vi "Controls.vi"() -> ()   [LabVIEW 2013]
uses:
  openfpgaref.8.6.ctl
  <vilib>/rvi/interface/nirviReadWriteControl/nirviReadWriteControl.xnode
  NiFpgaLv.dll
  <vilib>/Utility/error.llb/Error Cluster From Error Code.vi
  FPGA Bitfiles/UHR-FleezersInst_FPGATarget_UHR-Fleezers_Leonardo042018V4.lvbitx
  <vilib>/rvi/errors/niLvFpgaAdjustHostInterfaceError.vi
  <vilib>/gmath/NI_Gmath.lvlib
  <vilib>/gmath/statdist.llb/Exp Random.vi
  <vilib>/gmath/statdist.llb/Gamma Random.vi
  <vilib>/Platform/TimedLoop/XDataNode/wakeup.ctl
  <vilib>/Platform/TimedLoop/XDataNode/XDNodeRunTimeDep.lvlib
  <vilib>/Platform/TimedLoop/XDataNode/nitl_modes.ctl
  <vilib>/Platform/TimedLoop/XDataNode/timing_clust.ctl
  <vilib>/Platform/TimedLoop/XDataNode/XDataNode.xnode
  <vilib>/Utility/miscctls.llb/LVMinMaxIncTypeDef.ctl
panel:
  out "Current MCL (V)":dbl=5.657514378627918
  out "B factor":dbl=0.9916156324677038
  in  "Setpoint offset\nCorrection values":dbl[](array[numeric])=[0.024496601698410773, 0.024671186719617436, 0.024845771740824106, 0.025020356762030765, 0.02519494178323743, 0.025369526804444095, 0.025544111825650764, 0.025718696846857424, 0.025893281868064093, 0.026067866889270756, 0.026242451910477423, 0.026417036931684082, 0.02659162195289075, 0.026766206974097418, 0.02694079199530408, 0.027115377016510744, 0.027289962037717407, 0.027464547058924076, 0.02763913208013074, 0.027813717101337402, 0.027988302122544065, 0.02816288714375073, 0.028337472164957394, 0.02851205718616406, 0.028686642207370723, 0.028861227228577393, 0.02903581224978405, 0.029210397270990722, 0.029384982292197385, 0.02955956731340405, 0.02973415233461071, 0.029908737355817377, 0.030083322377024047, 0.03025790739823071, 0.030432492419437372, 0.030607077440644035, 0.0307816624618507, 0.030956247483057368, 0.03113083250426403, 0.0313054175254707, 0.03148000254667736, 0.03165458756788402, 0.03182917258909068, 0.03200375761029735, 0.032178342631504014, 0.03235292765271068, 0.03252751267391735, 0.03270209769512401, 0.03287668271633068, 0.033051267737537346, 0.033225852758744005, 0.03340043777995067, 0.03357502280115733, 0.033749607822364, 0.033924192843570664, 0.03409877786477733, 0.034273362885983996, 0.034447947907190656, 0.03462253292839732, 0.03479711794960398, 0.03497170297081065, 0.035146287992017314, 0.03532087301322398, 0.035495458034430646, 0.035670043055637306, 0.03584462807684397, 0.036019213098050645, 0.036193798119257305, 0.03636838314046397, 0.03654296816167063, 0.0367175531828773, 0.03689213820408396, 0.03706672322529063, 0.037241308246497296, 0.037415893267703955, 0.03759047828891062, 0.03776506331011729, 0.03793964833132395, 0.03811423335253061, 0.03828881837373728, 0.038463403394943946, 0.038637988416150605, 0.03881257343735727, 0.03898715845856393, 0.0391617434797706, 0.03933632850097726, 0.03951091352218393, 0.039685498543390596, 0.03986008356459726, 0.04003466858580393, 0.040209253607010595, 0.040383838628217254, 0.04055842364942392, 0.04073300867063058, 0.040907593691837246, 0.04108217871304391, 0.04125676373425058, 0.041431348755457245, 0.0416059337766639, 0.041780518797870564, 0.04195510381907723, 0.042129688840283896, 0.04230427386149057, 0.04247885888269723, 0.042653443903903895, 0.04282802892511056, 0.04300261394631722, 0.04317719896752389, 0.043351783988730554, 0.04352636900993721, 0.04370095403114388, 0.043875539052350546, 0.04405012407355721, 0.04422470909476388, 0.04439929411597054, 0.044573879137177204, 0.04474846415838387, 0.044923049179590537, 0.045097634200797196, 0.04527221922200386, 0.04544680424321053, 0.045621389264417195, 0.04579597428562386, 0.04597055930683052, 0.04614514432803718, 0.046319729349243846, 0.04649431437045051, 0.04666889939165718, 0.046843484412863845, 0.04701806943407051, 0.04719256456184452, 0.04736536676840916, 0.04753446267808822, 0.047696991448649737, 0.04784953848765512, 0.04799284096907562, 0.048127712917801824, 0.048257934523222495, 0.04838705366421733, 0.04851995197559876, 0.04865949840047511, 0.04880178465045004, 0.0489357994772595, 0.04905304538798107, 0.0491519464532862, 0.049234486275402736, 0.04930263064515607, 0.04935733149089569, 0.04939552771001872, 0.04941451823245213, 0.04941830757306315, 0.049410747020732684, 0.049392795273013504, 0.049367258833286985, 0.049339629147657244, 0.049311849604908836, 0.04928407006216041, 0.049256290519411994, 0.04922851097666357, 0.04920073143391515, 0.04917295189116673, 0.04914517234841831, 0.049117392805669895, 0.049089613262921473, 0.04906183372017306, 0.04903405417742463, 0.04900627463467622, 0.0489784950919278, 0.048950715549179374, 0.04892293600643097, 0.04889515646368254, 0.048867376920934125, 0.0488395973781857, 0.04881181783543728, 0.04878403829268886, 0.04875625874994044, 0.048728479207192026, 0.0487006996644436, 0.04867292012169519, 0.04864514057894676, 0.04861736103619835, 0.048589581493449926, 0.048561801950701505, 0.04853402240795309, 0.04850624286520466, 0.04847846332245625, 0.04845068377970783, 0.04842290423695941, 0.048395124694210985, 0.04836734515146257, 0.04833956560871415, 0.04831178606596573, 0.048284006523217314, 0.048256226980468886, 0.04822844743772048, 0.04820066789497206, 0.048172888352223636, 0.048145108809475215, 0.048117329266726794, 0.04808954972397837, 0.04806177018122996, 0.048033990638481544, 0.048006211095733116, 0.0479784315529847, 0.04795065201023628, 0.04792287246748786, 0.04789509292473944, 0.04786731338199102, 0.0478395338392426, 0.04781175429649418, 0.04778397475374576, 0.047756195210997346, 0.047728415668248925, 0.047700636125500503, 0.04767285658275208, 0.04764507704000366, 0.04761729749725524, 0.047589517954506826, 0.047561738411758404, 0.04753395886900998, 0.04750617932626157, 0.04747839978351315, 0.047450620240764727, 0.047422840698016305, 0.047395061155267884, 0.04736728161251948, 0.047339502069771056, 0.047311722527022634, 0.04728394298427421, 0.04725616344152579, 0.04722838389877737, 0.047200604356028956, 0.047172824813280535, 0.047145045270532114, 0.0471172657277837, 0.04708948618503528, 0.04706170664228686, 0.047033927099538436, 0.047006147556790015, 0.0469783680140416, 0.04695058847129318, 0.04692280892854476, 0.046895029385796344, 0.04686724984304792, 0.0468394703002995, 0.04681169075755108, 0.04678391121480266, 0.04675613167205424, 0.046728352129305824, 0.0467005725865574, 0.04667279304380899, 0.04664501350106057, 0.046617233958312146, 0.046589454415563725, 0.046561674872815303, 0.04653389533006689, 0.046506115787318475, 0.046478336244570054, 0.04645055670182163, 0.04642277715907321, 0.04639499761632479, 0.04636721807357637, 0.046339438530827955, 0.04631165898807953, 0.04628387944533112, 0.0462560999025827, 0.04622832035983428, 0.046200540817085856, 0.046172761274337434, 0.04614498173158901, 0.04611720218884059, 0.04608942264609218, 0.046061643103343757, 0.04603386356059534, 0.04600608401784692, 0.0459783044750985, 0.04595052493235008, 0.04592274538960166, 0.045894965846853236, 0.045867186304104815, 0.0458394067613564, 0.045811627218607986, 0.045783847675859565, 0.045756068133111144, 0.04572828859036272, 0.0457005090476143, 0.04567272950486588, 0.04564494996211747, 0.04561717041936905, 0.04558939087662063, 0.04556161133387221, 0.04553383179112379, 0.04550605224837537, 0.045478272705626946, 0.045450493162878525, 0.04542271362013011, 0.045394934077381696, 0.045367154534633275, 0.045339374991884854, 0.04531159544913643, 0.04528381590638801, 0.04525603636363959, 0.04522825682089117, 0.045200477278142755, 0.045172697735394333, 0.04514491819264592, 0.0451171386498975, 0.04508935910714908, 0.045061579564400656, 0.045033800021652234, 0.04500602047890381, 0.04497824093615539, 0.044950461393406985, 0.04492268185065856, 0.04489490230791014, 0.04486712276516172, 0.0448393432224133, 0.04481156367966488, 0.044783784136916464, 0.04475600459416805, 0.04472822505141963, 0.04470044550867121, 0.044672665965922786, 0.044644886423174365, 0.044617106880425944, 0.04458932733767752, 0.04456154779492911, 0.044533768252180694, 0.04450598870943227, 0.04447820916668385, 0.04445042962393543, 0.04442265008118701, 0.04439487053843859, 0.04436709099569017, 0.04433931145294175, 0.04431153191019333, 0.04428375236744492, 0.044255972824696496, 0.044228193281948075, 0.044200413739199654, 0.04417263419645123, 0.04414485465370281, 0.0441170751109544, 0.04408929556820598, 0.04406151602545756, 0.04403373648270914, 0.04400595693996072, 0.0439781773972123, 0.043950397854463884, 0.04392261831171546, 0.04389483876896704, 0.04386705922621863, 0.043839279683470206, 0.043811500140721785, 0.04378372059797336, 0.04375594105522494, 0.04372816151247652, 0.04370038196972811, 0.04367260242697968, 0.043644822884231264, 0.04361704334148285, 0.04358926379873443, 0.04356148425598601, 0.043533704713237587, 0.043505925170489165, 0.04347814562774075, 0.04345036608499233, 0.043422586542243916, 0.043394806999495494, 0.04336702745674707, 0.04333924791399865, 0.04331146837125023, 0.043283688828501816, 0.0432559092857534, 0.04322812974300498, 0.04320035020025656, 0.04317257065750814, 0.04314479111475972, 0.043117011572011296, 0.04308923202926288, 0.04306145248651446, 0.04303367294376604, 0.043005893401017625, 0.0429781138582692, 0.04295033431552078, 0.04292255477277236, 0.04289477523002394, 0.04286699568727552, 0.0428392161445271, 0.042811436601778684, 0.04278365705903027, 0.04275587751628185, 0.04272809797353343, 0.042700318430785006, 0.042672538888036585, 0.042644759345288163, 0.04261697980253975, 0.04258920025979133, 0.04256142071704291, 0.04253364117429449, 0.04250586163154607, 0.04247808208879765, 0.04245030254604923, 0.04242252300330081, 0.042394743460552387, 0.04236696391780398, 0.04233918437505556, 0.04231140483230714, 0.042283625289558716, 0.042255845746810294, 0.04222806620406188, 0.04220028666131346, 0.04217250711856504, 0.042144727575816616, 0.0421169480330682, 0.04208916849031978, 0.04206138894757136, 0.04203360940482294, 0.04200582986207452, 0.0419780503193261, 0.041950270776577675, 0.04192249123382926, 0.041894711691080846, 0.041866932148332425, 0.041839152605584004, 0.04181137306283558, 0.04178359352008716, 0.04175581397733874, 0.04172803443459032, 0.0417002548918419, 0.04167247534909349, 0.04164469580634507, 0.04161691626359665, 0.04158913672084823, 0.041561357178099806, 0.0415335776353514, 0.04150579809260298, 0.041478018549854556, 0.041450239007106135, 0.041422459464357714, 0.04139467992160929, 0.04136690037886087, 0.04133912083611246, 0.04131134129336403, 0.04128356175061562, 0.04125578220786719, 0.04122800266511878, 0.04120022312237036, 0.04117244357962194, 0.041144664036873516, 0.041116884494125094, 0.04108910495137668, 0.04106132540862826, 0.04103354586587984, 0.041005766323131417, 0.040977986780383, 0.04095020723763458, 0.04092242769488616, 0.04089464815213774, 0.04086686860938932, 0.0408390890666409, 0.04081130952389249, 0.04078352998114407, 0.040755750438395646, 0.040727970895647225, 0.040700191352898804, 0.04067241181015039, 0.040644632267401976, 0.04061685272465355, 0.04058907318190513, 0.04056129363915671, 0.04053351409640829, 0.04050573455365987, 0.04047795501091145, 0.040450175468163034, 0.04042239592541461, 0.0403946163826662, 0.04036683683991778, 0.04033905729716935, 0.040311277754420935, 0.040283498211672514, 0.0402557186689241, 0.04022793912617567, 0.04020015958342725, 0.040172380040678836, 0.04014460049793042, 0.040116820955182, 0.04008904141243358, 0.04006126186968516, 0.04003348232693674, 0.04000570278418832, 0.03997792324143991, 0.03995014369869149, 0.039922364155943066, 0.039894584613194645, 0.03986680507044622, 0.0398390255276978, 0.03981124598494939, 0.03978346644220096, 0.039755686899452546]
  in  "Negate offset difference":bool
  in  "Target Force (pN)":dbl=10.5
  out "Trap X (AI1)":T1={"Trap 1"=0.030792236328125, "Trap 2"=-0.011322021484375}
  out "Trap X AI1 (DMA)":T2={"Set 1"=0.030731201171875, "Set 2"=-0.0113525390625}
  in  "Pump 1 contents":string="Top: DNA beads" caption="contents"
  in  "All Pump Parameters":T3={"Pump 1"={"Diameter (mm)"=4.61, "Units"=4.0, "Volume"=100.0, "Rate"=50.0}, "Pump 2"={"Diameter (mm)"=4.61, "Units"=3.0, "Volume"=0.0, "Rate"=0.0}, "Pump 3"={"Diameter (mm)"=4.61, "Units"=4.0, "Volume"=100.0, "Rate"=250.0}}
  in  "Pump write delay (ms)":dbl=300.0
  in  "Save scans":bool=TRUE
  out "MCL Scanning":bool
  in  "T1 alpha_x (nm/V)":dbl=701.8425766517444 step=10.0 format="%#_3g"
  in  "T2 alpha_x (nm/V)":dbl=806.869454518421 step=10.0 format="%#_3g"
  in  "T1 kappa_x (pN/nm)":dbl=0.1608167093260824 min=0.0 step=0.001 format="%#_2g"
  in  "T2 kappa_x (pN/nm)":dbl=0.13871102209446912 min=0.0 step=0.001 format="%#_2g"
  in  "T1 offset_x (mV)":dbl=44.132512662199076 format="%#_2g"
  in  "T2 offset_x (mV)":dbl=-16.403354316809207 format="%#_2g"
  in  "Freq switch delay":u16=9
  in  "Swap F1 and F2":bool
  in  "Amp switch delay":u16=4
  in  "Phase offset method":u8=3
  in  "Phase increment trap 1":fxp<+/-,64,32>
  in  "Phase increment trap 2":fxp<+/-,64,32>
  in  "RF phase reset before cycles":bool
  out "Initial delta (MHz)":dbl=20.0
  in  "AOM X Cal (nm/MHz)":dbl=174.0
  in  "Invert APD Gate":bool caption="Invert Gate"
  in  "APD Gate ON Count":u32=150 caption="Gate ON Count"
  in  "APD Gate OFF Count":u32=450 caption="Gate OFF Count"
  in  "APD Gate":enum32{"ON", "OFF", "Interlace"}(radio)=enum."Interlace"
  in  "APD Integration Time (s)":dbl=0.01 caption="Integration Time (s)"
  in  "APD 1 AO Mult.":i16=1 min=1
  in  "APD 2 AO Mult.":i16=1 min=1
  in  "Phase Adj. (APD Acq)":i16=20
  in  "Phase Adj. (APD 2 Gate)":i16=20
  in  "Phase Adj. (APD 1 Gate)":i16=20
  in  "Green FB Gains":T4={"proportional gain (Kc)"=10, "integral gain (Kc*Ts/Ti)"=5, "derivative gain (Kc*Td/Ts)"=0}
  in  "Current When FB OFF (%)":dbl=10.0 min=0.0 max=100.0 step=1.0
  in  "Green int current ON count adj":u32=150
  in  "Green FB Setpoint (mV)":dbl=100.0
  in  "PID gains":T4={"proportional gain (Kc)"=0, "integral gain (Kc*Ts/Ti)"=5, "derivative gain (Kc*Td/Ts)"=0}
  in  "DIO count 1 (ticks)":u32=200
  in  "DIO count 2 (ticks)":u32=200
  in  "DIO count 3 (ticks)":u32=200
  in  "BD 1 Amplitude 1 (%)":dbl=40.0 min=0.0 max=75.0 step=1.0
  in  "BD 1 Amplitude 2 (%)":dbl=42.0 min=0.0 max=75.0 step=1.0
  in  "BD 1 Amplitude 3 (%)":dbl min=0.0 max=75.0 step=1.0
  in  "BD 2 Amplitude 1 (%)":dbl min=0.0 max=75.0 step=1.0
  in  "BD 2 Amplitude 2 (%)":dbl min=0.0 max=75.0 step=1.0
  in  "BD 2 Amplitude 3 (%)":dbl min=0.0 max=75.0 step=1.0
  out "X RF Amplitude Limits (%)":T5={"Minimum"=0.0, "Maximum"=75.0, "Increment"=1.0}
  out "Y RF Amplitude Limits (%)":T5={"Minimum"=0.0, "Maximum"=75.0, "Increment"=1.0}
  out "Feedback overload":bool
  out "APD 1 Rate (Hz)":dbl format="%#_3p"
  out "AI labels":string[](array[string])=["T1 Y", "T1 X", "T1 Sum", "T2 Y", "T2 X", "T2 Sum", "T1 FB X", "T2 FB Sum", "T2 FB X", "T2 FB Sum", "PSD Y", "PSD X", "PSD Sum"]
  out "Bead Mean (nm)":dbl=13.506045465071283 caption="Mean (nm)" format="%0.2f"
  in  "AI Count (ticks)":u32=200
  in  "N sets to save":u32=200 caption="N Sets"
  out "APD Int. Count":u32=400000 format="%.0p"
  in  "Scale intensities":bool
  in  "Scale factor":dbl=0.25
  in  "MCL Tracking":bool
  out "Zero MCL x position":dbl=5.6547922360429315
  out "Zero T1 position":dbl=70.0
  in  "Read setpoint correction\nfile":bool
  in  "Setpoint correction\noffset file":path
  in  "Raster target force (pN)":dbl=10.0
  in  "Trap Pos FB Int Count":u16=100
  in  "Trap Pos. FB Out Scale 2^n":u8=23 caption="Action Scale"
  in  "Set SP to Reading":bool
  in  "Set SP Using...":bool
  in  "Simulate stepping":bool
  in  "Step size (nm)":dbl min=0.0
  in  "Backtrack probability":dbl min=0.0 max=1.0
  in  "Mean dwell time (s)":dbl=0.001 min=0.001
  in  "Distribution":enum16{"uniform", "Exponential", "Gamma2"}(ring)
  out "Step taken":dbl
  in  "Number of steps":i32
  out "Step duration":dbl
  in  "Trap Pos FB SP":fxp<+/-,16,1>=0.231353759765625 caption="Setpoint"
  in  "Trap Pos. FB Range":T6={"output high"=0.999969482421875, "output low"=-1.0}
  in  "Trap Pos. FB Gains":T7={"proportional gain (Kc)"=20.0, "integral gain (Kc*Ts/Ti)"=3.0, "derivative gain (Kc*Td/Ts)"=0.0} {"proportional gain (Kc)" format="%.11g"; "integral gain (Kc*Ts/Ti)" format="%.11g"; "derivative gain (Kc*Td/Ts)" format="%.11g"}
  in  "Trap Pos. FB Mult Factor":i64=8388608
  in  "Trap Pos. FB Offset Factor":i64
  in  "Trap Pos FB Negate Action":bool=TRUE
  in  "Trap Pos FB Monitor\nT1 or T2":bool
  in  "Trap Pos. AI1 X Pre-scale":u16
  in  "Diff. FB.":bool=TRUE
  in  "Negate Diff?":bool
  in  "Trap Pos. FB ON":bool
  in  "Reset Trap Pos. FB":bool
  out "Pump 1 cont disp":string="Right: DNA beads "
  out "Pump 3 cont disp":string="Left: ADig beads"
  in  "Flip Green Filter":bool
  in  "Shunt:":bool
  in  "Inject Bottom":bool
  in  "Flush Center Ch Volume (uL)":dbl=15.0
  in  "Flush Center Ch Rate (ul/m)":dbl=100.0
  in  "Total Volume\nFlushed (uL)":dbl
  in  "Inject Valve B":bool caption="Inject Pump 2\n(Flush Center)"
  in  "Ch 3 Inject Volume (uL)":dbl=100.0
  in  "Ch 3 Inject Rate (ul/h)":dbl=250.0
  in  "Pump 3 contents":string="Bottom: ADig beads" caption="contents"
  in  "Chemyx Syringe Pump Serial Port":refnum<visa-resource-name>="ASRL3::INSTR"
  in  "Main:":bool caption="Inject Pump 3"
  in  "Ch 2 Inject Volume (uL)":dbl=100.0
  in  "Ch 1 Inject Rate (ul/h)":dbl=50.0
  in  "Pump pause delay (ms)":u32
  in  "Inject Top:":bool caption="Inject Pump 1"
  in  "Index":dbl=43.0 caption="Save File Index" min=1.0 step=1.0
  out "Save file name":path=path "I:/Data/160525/160525_043.dat"
  out "Save index":dbl=43.0
  in  "Continuous AOD Scanning":bool caption="Continuous Scanning"
  in  "Abort AOD Scan":bool caption="Abort Scan"
  in  "Phase adjust (MCL)":i16 caption="Phase adjust"
  in  "- phase (MCL)":bool
  in  "+ phase (MCL)":bool
  in  "Update Count (MCL)":u32=600
  in  "Abort MCL Scan":bool
  out "Read cal error":errorcluster
  in  "Read Cal":bool
  out "Offset file step size":dbl=0.1
  in  "Offset Values":T8={"Trap 1X offset"=array[500 elements], "Trap 2X offset"=array[500 elements]}
  in  "Auto read offset\ncorrection":bool=TRUE
  out "Data points/scan (f+b)":dbl=240.0 caption="points/scan (f+b)"
  out "Data points/scans (MCL)":dbl=4800.0 caption="Data points/scans"
  in  "Number of scans (MCL)":u64=1 caption="Scans"
  out "Cycles/step (MCL)":u64=2000 caption="Cycles/step" format="%.0p"
  out "N sets should be saved (MCL)":dbl=160.0 caption="N sets should be saved"
  out "Time/f+b scan (s) (MCL)":dbl=2.4 caption="Time/scan (s)"
  out "Desired Scan Incr (V)":dbl=0.14102564102564102
  out "Actual Incr. int (MCL)":i16=462 caption="Incr. int"
  out "Desired incr (int)":dbl=462.098717948718
  in  "N APD Samp/step":dbl=3.0
  in  "Scan Range (V)\n(of steps)":dbl=3.5
  in  "2D or 1D Scan":bool=TRUE
  in  "Fast Scan Dir":bool=TRUE
  in  "Continuous MCL Scanning":bool caption="Cont. Scanning"
  out "Total Time (s) 2":dbl=48.0
  out "Scan steps (AOD)":u64=2000
  out "Data points/scan (f/b)":dbl=2664000.0
  out "Data points/scans":dbl=2664000.0
  in  "Number of F/B Scans (AOD)":u16=1 min=1
  out "Cycles/step (AOD)":u64=666 format="%.3p"
  out "N sets should be saved":dbl=133.2
  out "Time/Scan (s) (AOD)":dbl=19.98 format="%#_2p"
  out "Scan Increment (MHz)":dbl=-0.0050025012506253125
  out "Incr. int (AOD)":i64=-5670036101
  out "Scan Range (MHz)":dbl=-10.0
  out "Final freq. (MHz)":dbl=60.0
  in  "Scan BD":bool=TRUE
  out "Initial freq. (MHz)":dbl=70.0
  out "Final delta (MHz)":dbl=30.0
  out "Final sep (nm)":dbl=1590.0
  out "Initial sep (nm)":dbl=360.0
  in  "Step Size (nm)":dbl=1.0
  in  "Scan Range (nm)":dbl=1683.3000000000002
  in  "Trap 2 Bead Size (nm)":dbl=2100.0
  in  "Trap 1 Bead Size (nm)":dbl=2100.0
  in  "Scan Speed (nm/s)":dbl=100.0
  out "Time to Finish All (min)":dbl=0.666 format="%#_2p"
  in  "GI Frequency, ON count":u32=150 min=1 step=1
  in  "Green FB Count":u32=600
  in  "GI Frequency, OFF count":u32=450 min=1 step=1
  out "APD Acq Rate (Hz)":dbl=100.0 caption="Rate (Hz)"
  in  "+ phase (Green FB)":bool
  in  "- phase (Green FB)":bool
  in  "Phase adj. (Green FB)":i16=10
  in  "Phase adj. (GI) 2":i16=20
  in  "+ phase (GI) 2":bool
  in  "- phase (GI) 2":bool
  in  "+ phase (GI)":bool
  in  "- phase (GI)":bool
  in  "Phase adj. (GI)":i16=5
  in  "+ phase (APD Acq)":bool
  in  "- phase (APD Acq)":bool
  in  "- phase (APD 2 Gate)":bool
  in  "+ phase (APD 2 Gate)":bool
  in  "- phase (APD 1 Gate)":bool
  in  "+ phase (APD 1 Gate)":bool
  in  "Invert GI":bool
  in  "AI2 to Setpoint":cluster{"Set 1":bool, "Set 2":bool}
  in  "Trap Intensity\nSetpoints (V)":cluster{"Set 1":dbl, "Set 2":dbl}={"Set 1"=5.0, "Set 2"=5.0}
  out "AI2 (V)":cluster{"Set 1":dbl, "Set 2":dbl}={"Set 1"=3.087557603686636, "Set 2"=2.914212469862972}
  in  "Reset Feedback":cluster{"Set 1":bool, "Set 2":bool}
  in  "Interlace":bool=TRUE
  in  "Number Interlace Sets":u8=3 min=1 max=3
  in  "Not-Interlacing Set":enum32{"Set 1", "Set 2", "Set 3"}(radio)
  out "Total Counts (ticks)":u32=600
  in  "Trap 1 (ON/OFF)":bool=TRUE
  in  "Trap 2 (ON/OFF)":bool=TRUE
  in  "Saved AOD Raster Scan Parameter Sets":T9(array[cluster])=[{"Scan Range AOD (nm) 2"=500.0, "Step Size AOD (nm) 2"=1.0, "Scan Speed AOD (nm/s) 2"=100.0, "Number of scans (AOD) 2"=1, "Label"="offset curve"}, {"Scan Range AOD (nm) 2"=1000.0, "Step Size AOD (nm) 2"=1.0, "Scan Speed AOD (nm/s) 2"=100.0, "Number of scans (AOD) 2"=1, "Label"="hp raster check"}, {"Scan Range AOD (nm) 2"=6.8, "Step Size AOD (nm) 2"=0.34, "Scan Speed AOD (nm/s) 2"=0.34, "Number of scans (AOD) 2"=1, "Label"="3.4 kbp - 1 bp steps"}]
  in  "Load parameters":bool
  in  "Trap 1 ON":bool=TRUE
  in  "Trap 2 ON":bool=TRUE
  in  "Trap 3 ON":bool
  in  "Trap ON/OFF X or Y Amp?":bool=TRUE
  in  "Feedback On/Off":cluster{"Set 1":bool, "Set 2":bool}={"Set 1"=TRUE, "Set 2"=TRUE}
  in  "All FB On/Off":bool
  in  "Delayed Interlace Start":bool
  in  "Delay to Interlace (s)":dbl
  in  "Round T2 X":bool caption="Round"
  in  "Round T1 X":bool caption="Round"
  in  "Oscillate Set 2":bool
  in  "Middle freq for \nsymmetric (MHz)":dbl=78.0
  in  "T2 for asymmetric\n(MHz)":dbl=85.0
  in  "Symmetric manual \ntrap motion":bool
  in  "Dynamic Force FB":bool=TRUE
  in  "Phase adj. (AI1)":i16
  in  "- phase (AI1)":bool
  in  "+ phase (AI1)":bool
  in  "Adjust Scale\nto Mean":bool
  in  "Above (kHz)":dbl=2.0
  in  "Below (kHz)":dbl=0.5
  in  "Rescale on Mean":bool
  in  "Amplitude (nm)":dbl=1.0
  out "AI rate (Hz)":dbl=200000.0 format="%#_6p"
  out "Ave. Rate (Hz)":dbl=200000.0 format="%#_6p"
  out "Ave. Period (s)":dbl=5e-06 format="%#_6p"
  out "Data Rate (Hz)":dbl=66666.66666666667 caption="Trap Data Rate (Hz)" format="%#_3p"
  out "Data Period (s)":dbl=1.4999999999999999e-05 caption="Trap Data Period (s)" format="%#_6p"
  in  "Sets to FIFO (Traps)":T10={"Set 1"=TRUE, "Set 2"=TRUE, "Set 3"=FALSE}
  out "Save Data Rate (Hz)":dbl=133.33333333333334 caption="Rate (Hz)" format="%#_6p"
  out "Save Data Period (s)":dbl=0.0075 caption="Period (s)" format="%#_6p"
  in  "N Acq Sets (Traps + Fl.)":i16=3
  out "# Samples/channel":u32=40000 format="%.0p"
  out "Trap AI Elements/DMA read":u32=320000 format="%.0p"
  out "DMA Update Period (s)":dbl=0.3
  out "APD Samples/FIFO Acq.":dbl=30.0
  out "Total Time (s)":dbl=60.0
  in  "# Samples/trap":u32=20000 format="%.0p"
  out "APD Elements/DMA read":u32=60
  out "Trap Sets":u32=2
  out "FPGA Averaging":bool
  out "Counts/DMA":dbl=12000000.0 format="%#_6p"
  out "Trap Pos Elements/DMA read":u32=120000 format="%.0p"
  out "error out 2":errorcluster
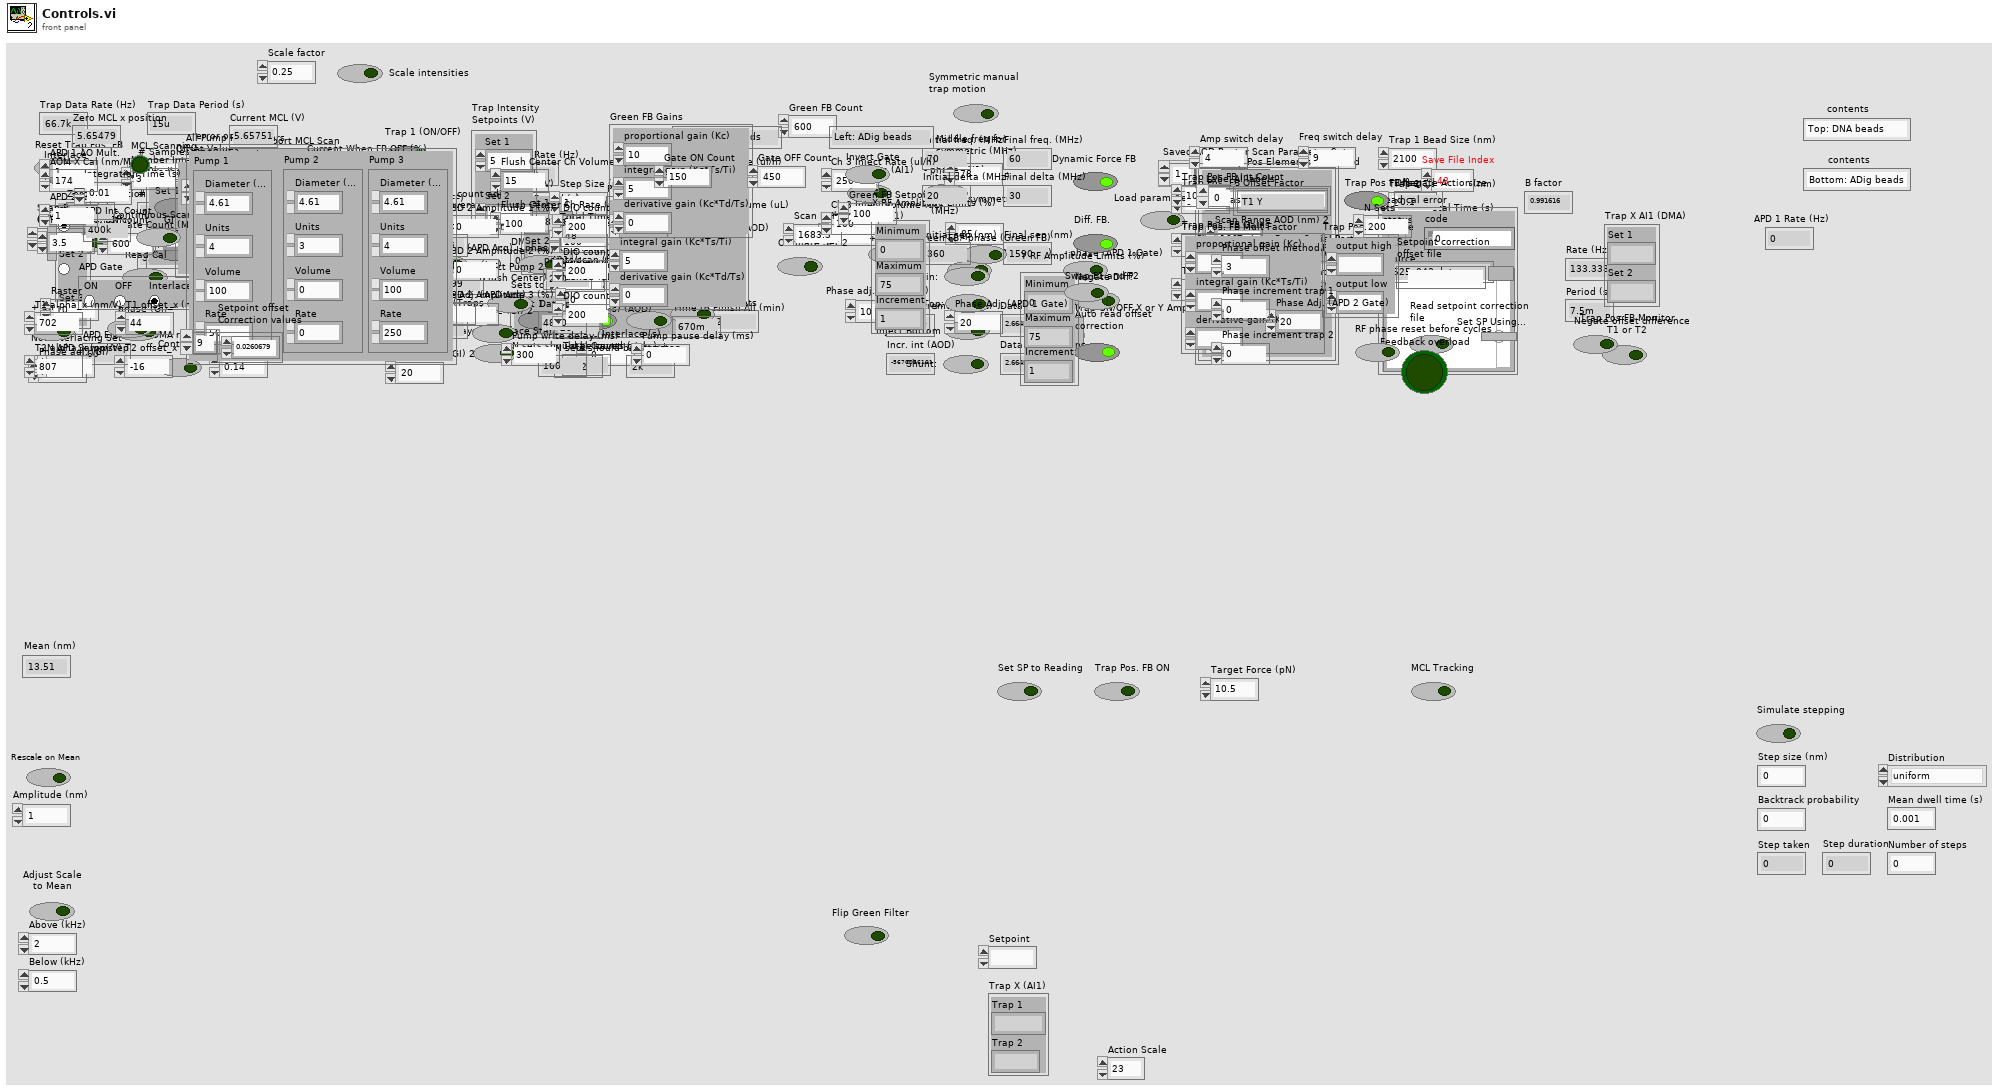
[diagram p1: front panel]
types:
  T1 = cluster{"Trap 1":fxp<+/-,16,1>, "Trap 2":fxp<+/-,16,1>}
  T2 = cluster{"Set 1":fxp<+/-,16,1>, "Set 2":fxp<+/-,16,1>}
  T3 = cluster{"Pump 1":cluster{"Diameter (mm)":dbl, "Units":dbl, "Volume":dbl, "Rate":dbl}, "Pump 2":cluster{"Diameter (mm)":dbl, "Units":dbl, "Volume":dbl, "Rate":dbl}, "Pump 3":cluster{"Diameter (mm)":dbl, "Units":dbl, "Volume":dbl, "Rate":dbl}}
  T4 = cluster{"proportional gain (Kc)":i16, "integral gain (Kc*Ts/Ti)":i16, "derivative gain (Kc*Td/Ts)":i16}
  T5 = typedef "LVMinMaxIncTypeDef.ctl" = cluster{"Minimum":dbl, "Maximum":dbl, "Increment":dbl}
  T6 = cluster{"output high":fxp<+/-,16,1>, "output low":fxp<+/-,16,1>}
  T7 = cluster{"proportional gain (Kc)":fxp<+/-,16,8>, "integral gain (Kc*Ts/Ti)":fxp<+/-,16,8>, "derivative gain (Kc*Td/Ts)":fxp<+/-,16,8>}
  T8 = cluster{"Trap 1X offset":dbl[], "Trap 2X offset":dbl[]}
  T9 = cluster{"Scan Range AOD (nm) 2":dbl, "Step Size AOD (nm) 2":dbl, "Scan Speed AOD (nm/s) 2":dbl, "Number of scans (AOD) 2":u16, "Label":string}[]
  T10 = cluster{"Set 1":bool, "Set 2":bool, "Set 3":bool}
  T11 = typedef "XDNodeRunTimeDep.lvlib/timing_clust.ctl" = cluster{"Expected End [f-1]":u64, "Actual End [f-1]":u64, "Finished Late? [f-1]":bool, "Expected End [i-1]":u64, "Actual End [i-1]":u64, "Finished Late? [i-1]":bool, "Expected Start [i]":u64, "Actual Start [i]":u64, "Expected Start [f]":u64, "Actual Start [f]":u64, "Source Name":string, "Structure Name":string, "Period":i64, "Deadline":i64, "Offset":i64, "Start":i64, "Priority":i32, "Timeout":i32, "Mode":T12, "Wakeup Reason":T13, "Error":errorcluster, "Source Type":string, "Secondary Source Type":string, "Global End Time":u64, "Global Start Time":u64, "Frame Duration":u64, "Iteration Duration":u64, "Assigned CPU":i32, "I/O Scan Engine Mode":u32}
  T12 = typedef "XDNodeRunTimeDep.lvlib/nitl_modes.ctl" = enum32{"No Change", "Process missed periods, maintain original phase", "Discard missed periods, maintain original phase", "Process missed periods, ignore original phase", "Discard missed periods, ignore original phase"}
  T13 = typedef "XDNodeRunTimeDep.lvlib/wakeup.ctl" = enum32{"Normal", "Aborted", "Asynchronous wakeup", "Timing source error", "Timed loop error", "Timeout"}
  T14 = enum16{"CONNECT", "INITIALIZE VALVES", "DISCONNECT", "MOVE VALVE"}
  T15 = enum16{"open", "replace", "create", "open or create", "replace or create", "replace or create with confirmation"}
  T16 = enum16{"big-endian, network order", "native, host order", "little-endian"}
  T17 = typedef "openfpgaref.8.6.ctl" = refnum<k20>
  T18 = cluster{"Scan Range AOD (nm) 2":dbl, "Step Size AOD (nm) 2":dbl, "Scan Speed AOD (nm/s) 2":dbl, "Number of scans (AOD) 2":u16, "Label":string}
  T19 = cluster{"[0]":dbl, "[1]":dbl, "[2]":dbl, "[3]":dbl, "[4]":dbl, "[5]":dbl}
  T20 = cluster{"Diameter (mm)":dbl, "Units":dbl, "Volume":dbl, "Rate":dbl}
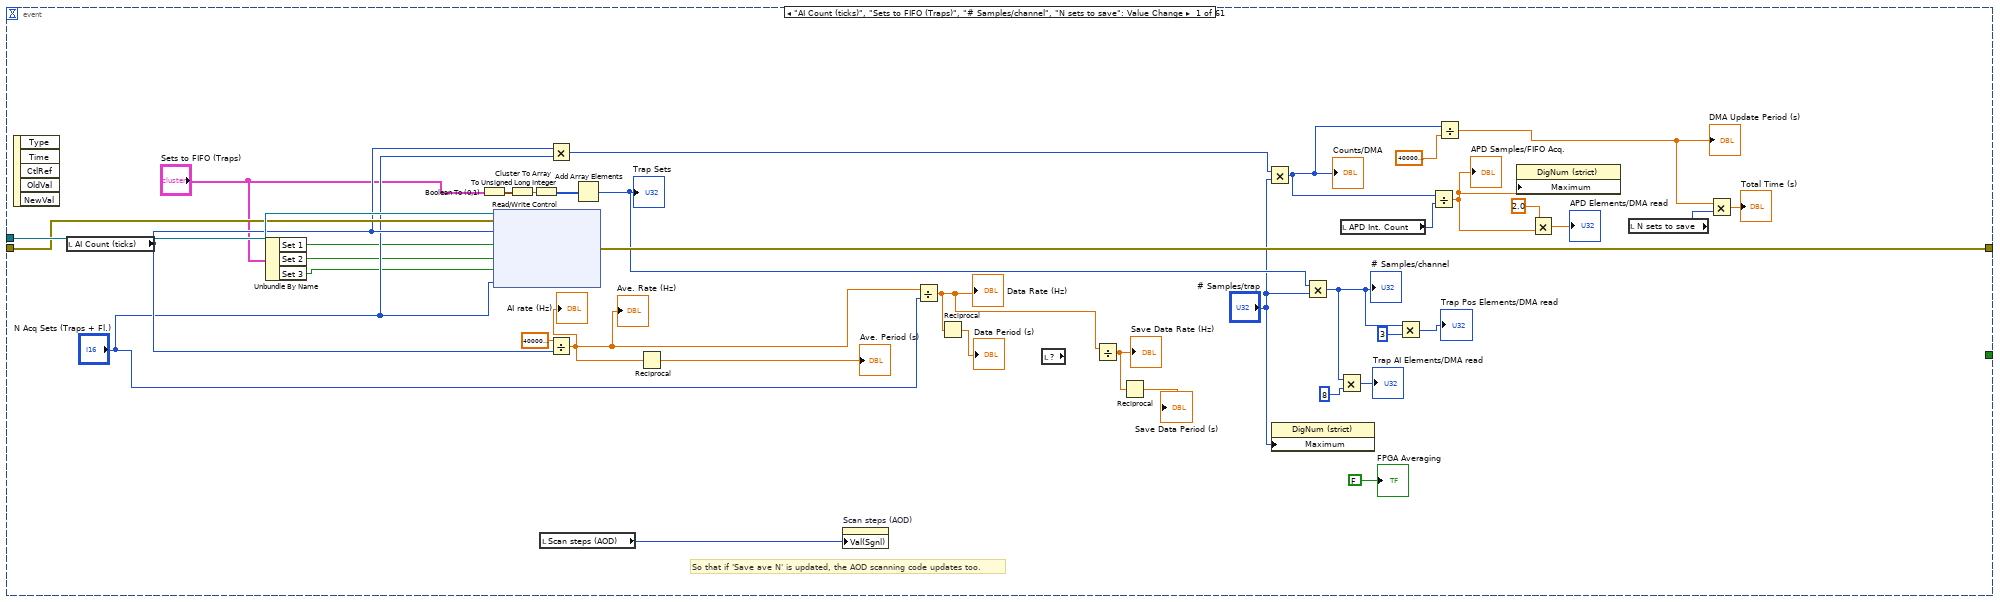
[diagram p2: hidden frame]
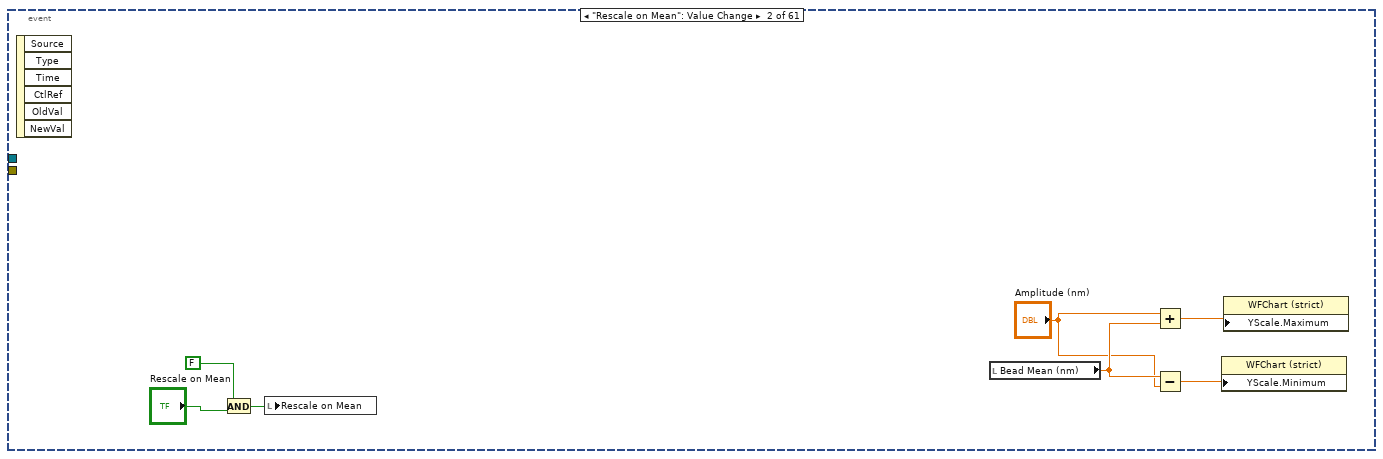
[diagram p3: hidden frame]
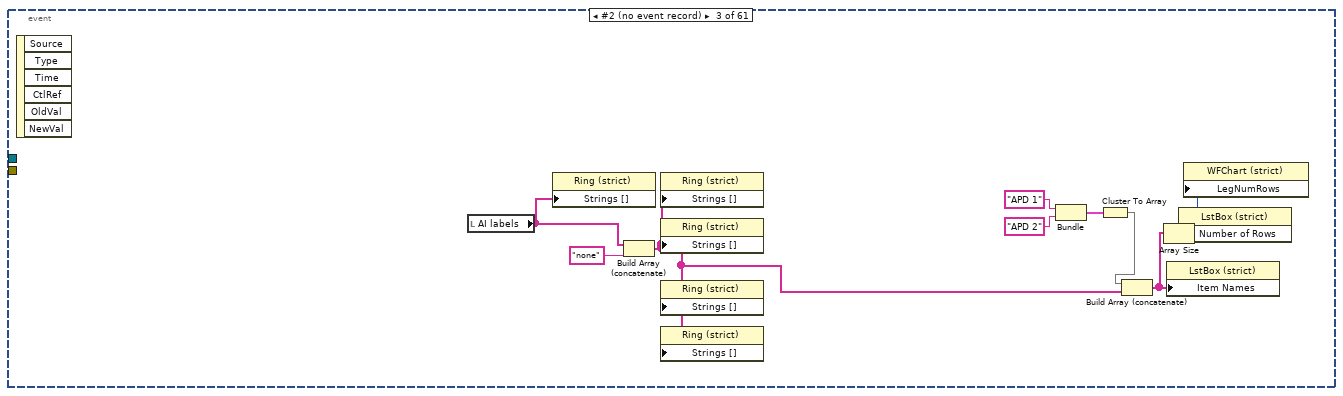
[diagram p4: hidden frame]
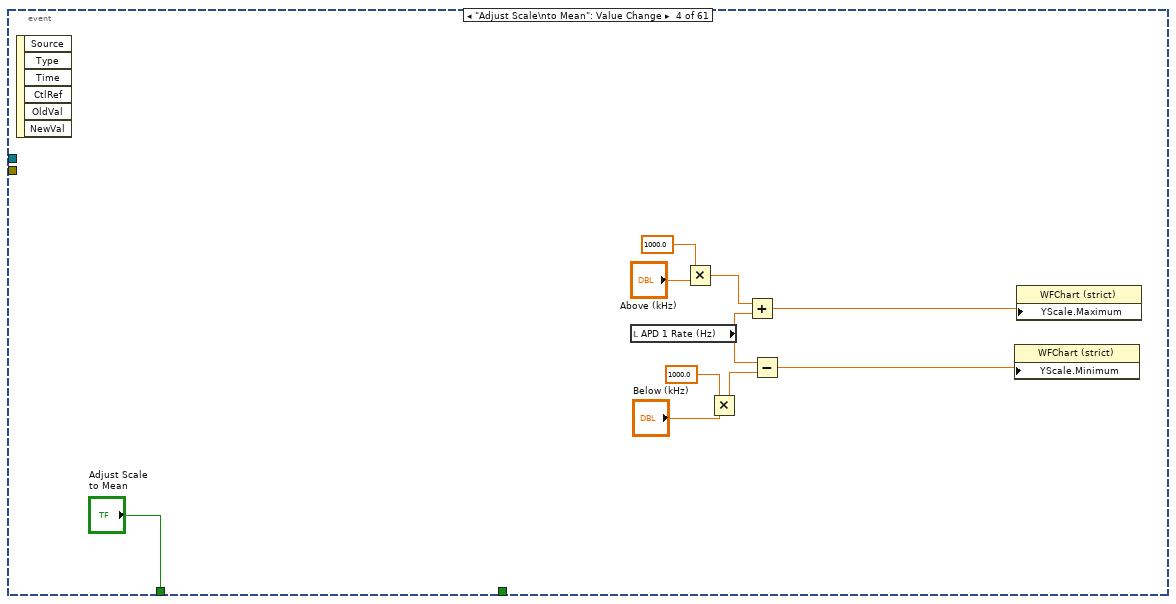
[diagram p5: hidden frame]
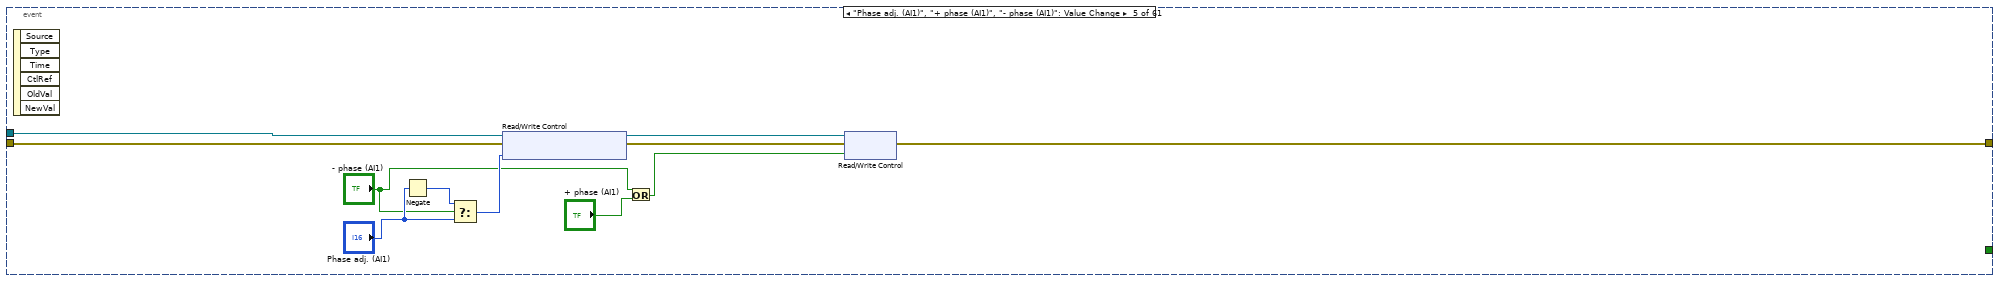
[diagram p6: hidden frame]
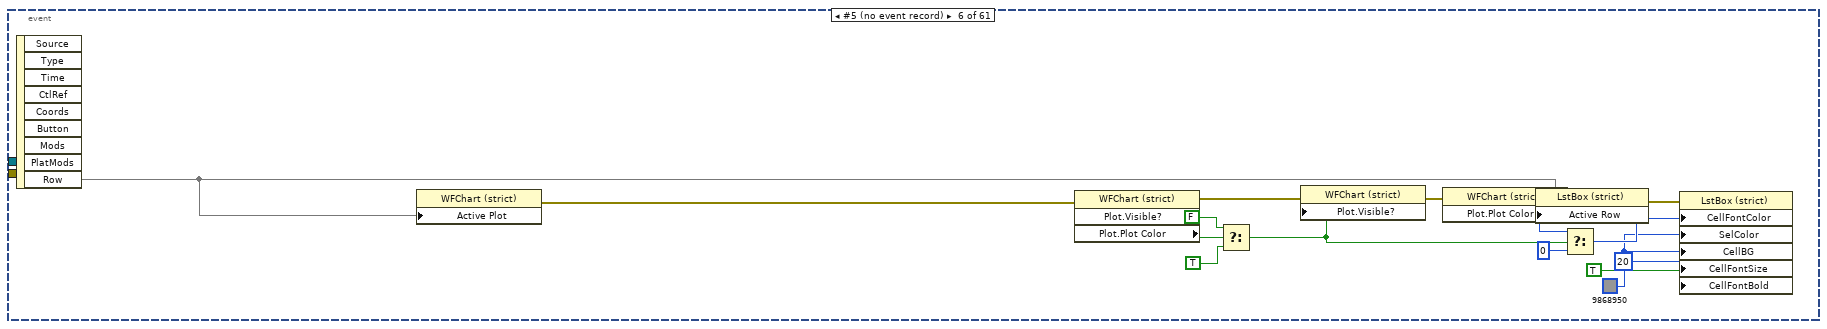
[diagram p7: hidden frame]
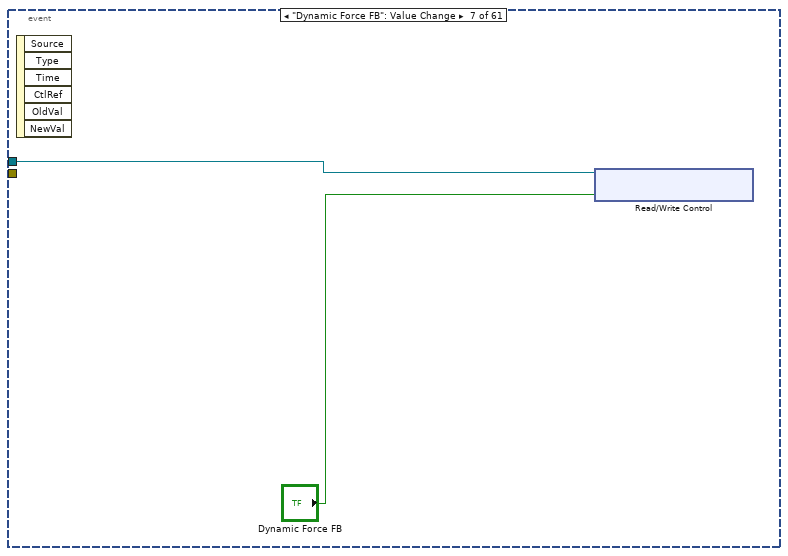
[diagram p8: hidden frame]
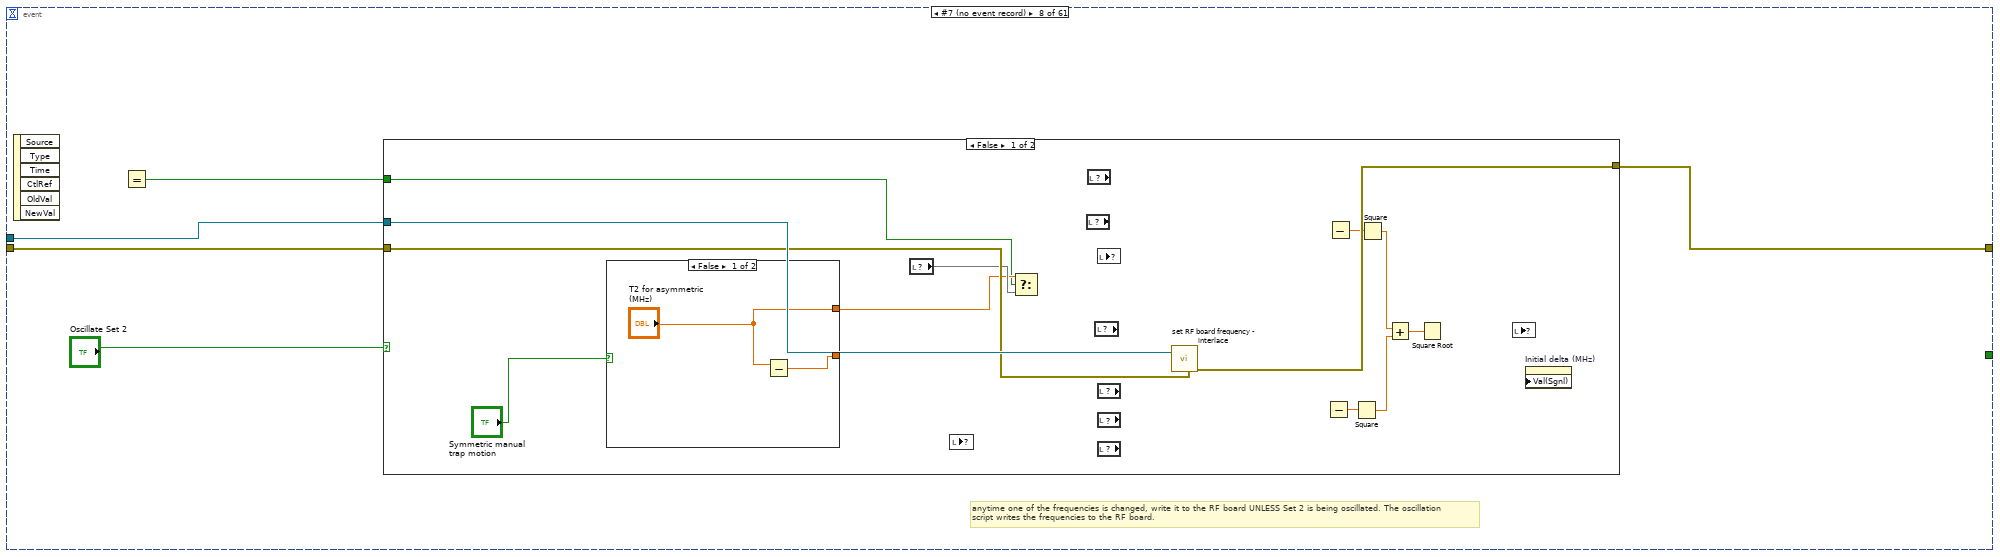
[diagram p9: hidden frame]
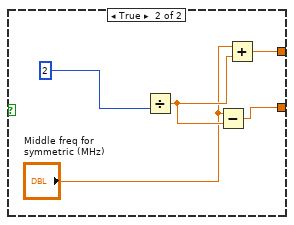
[diagram p10: hidden frame]
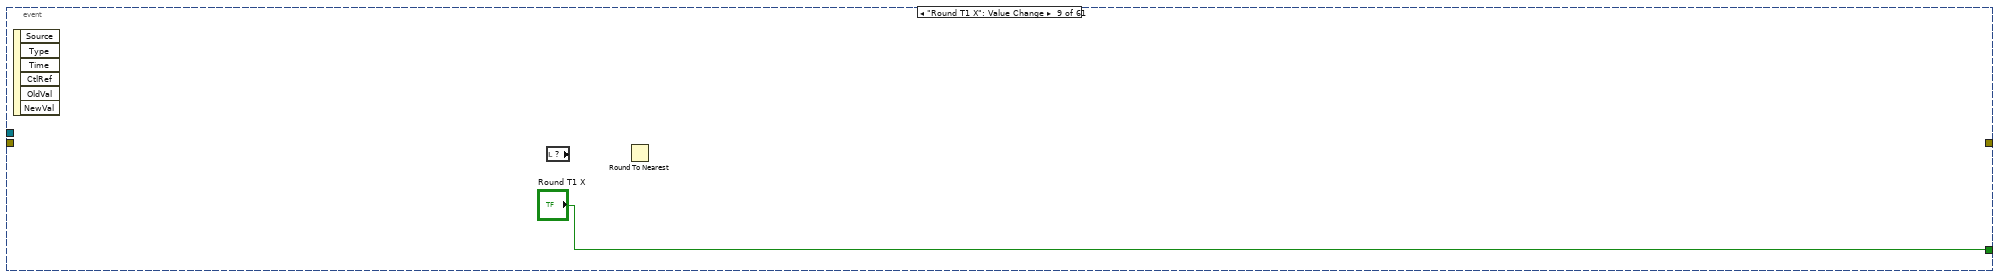
[diagram p12: hidden frame]
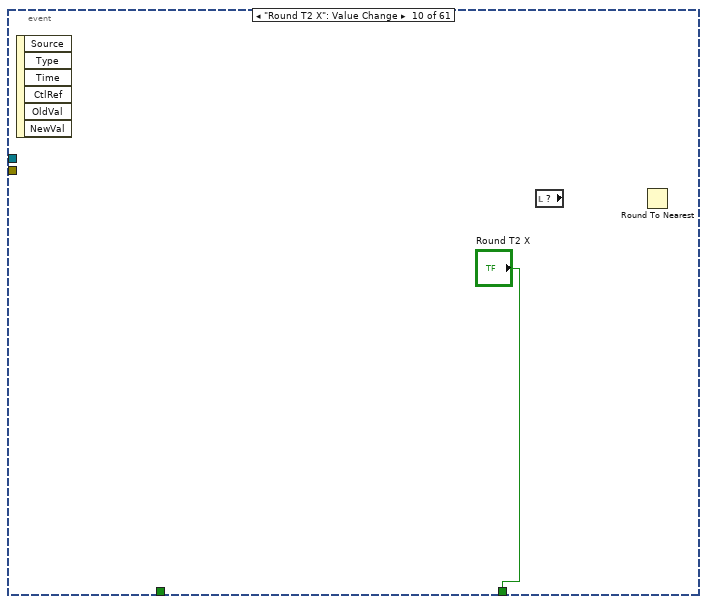
[diagram p13: hidden frame]
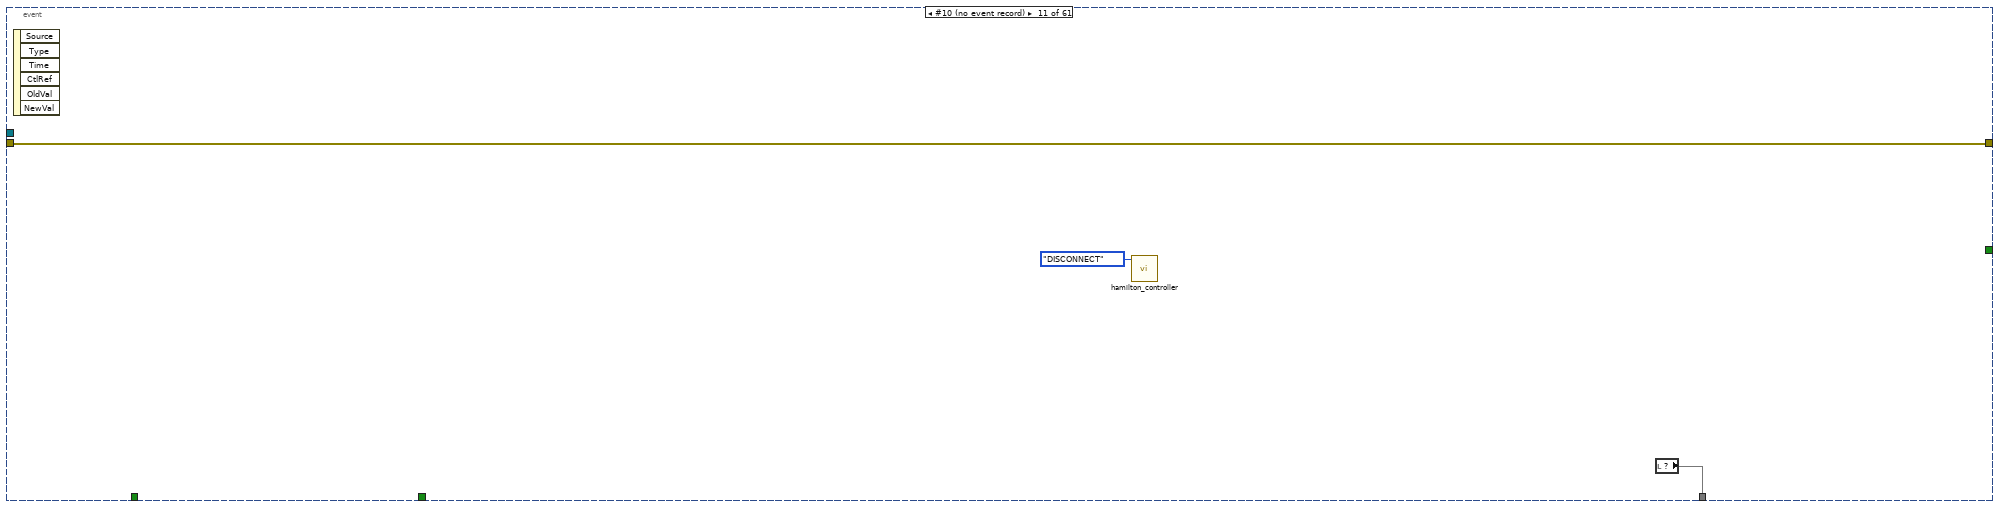
[diagram p14: hidden frame]
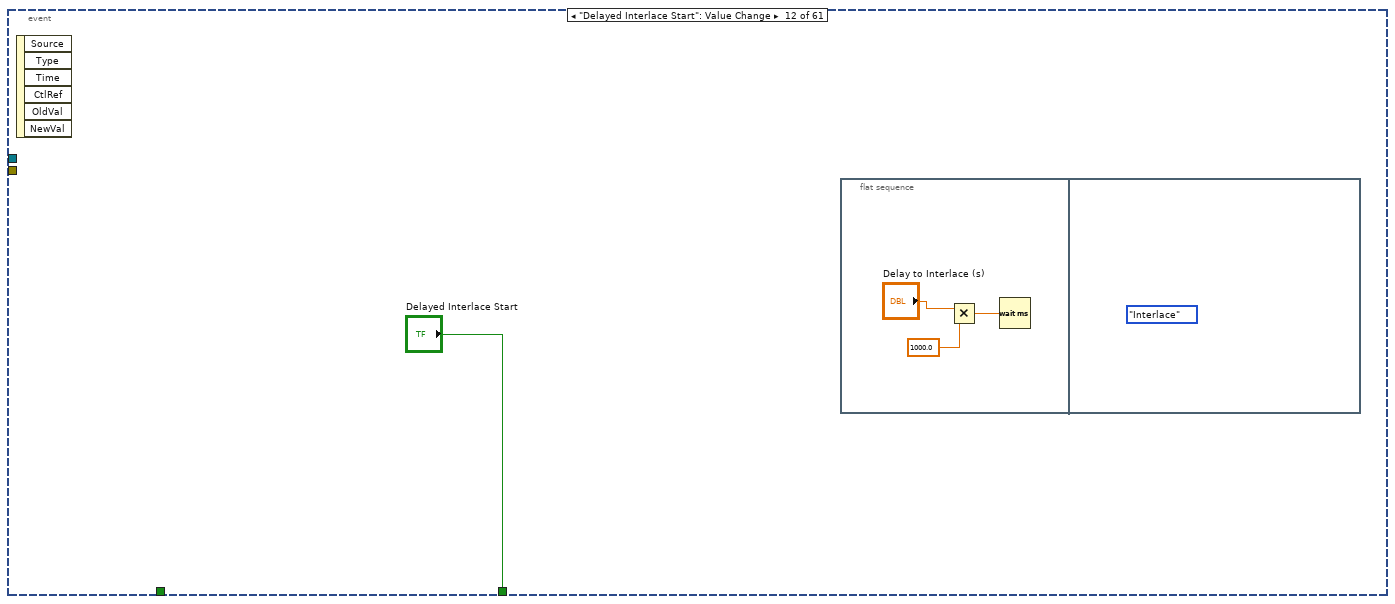
[diagram p15: hidden frame]
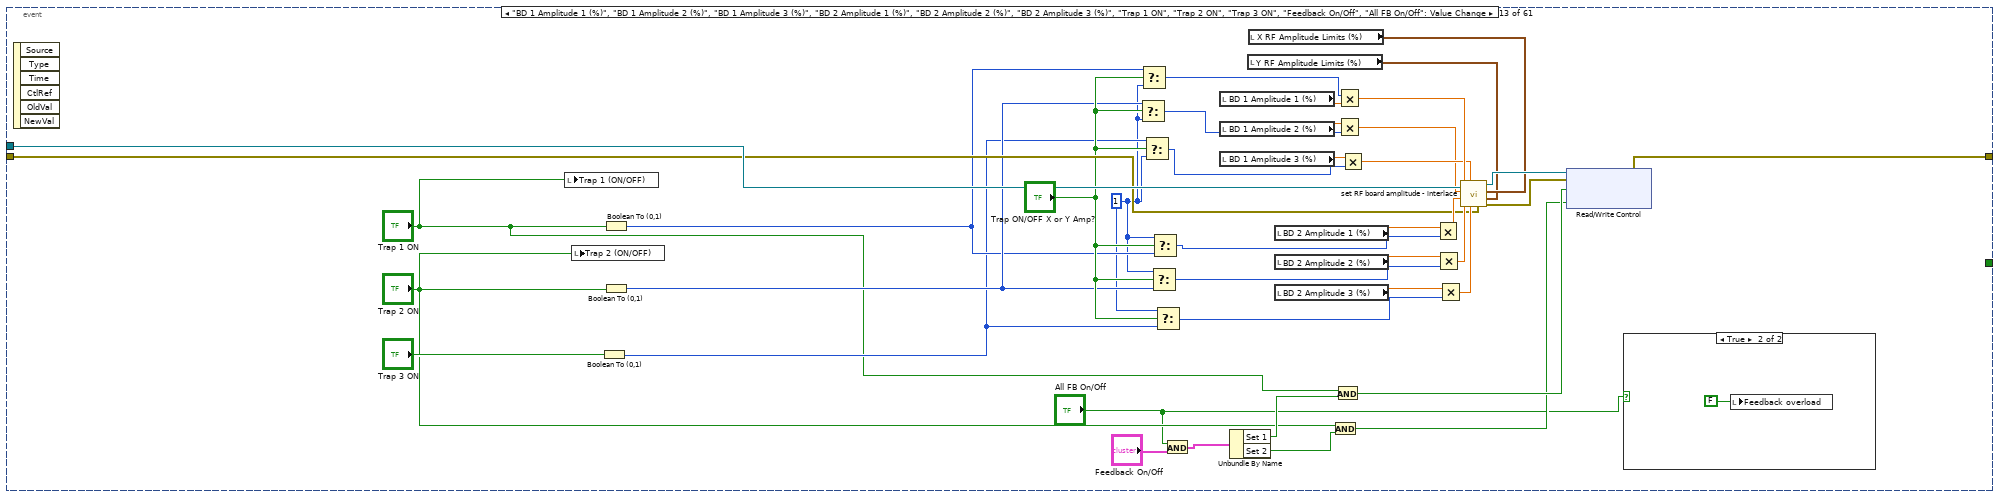
[diagram p16: hidden frame]
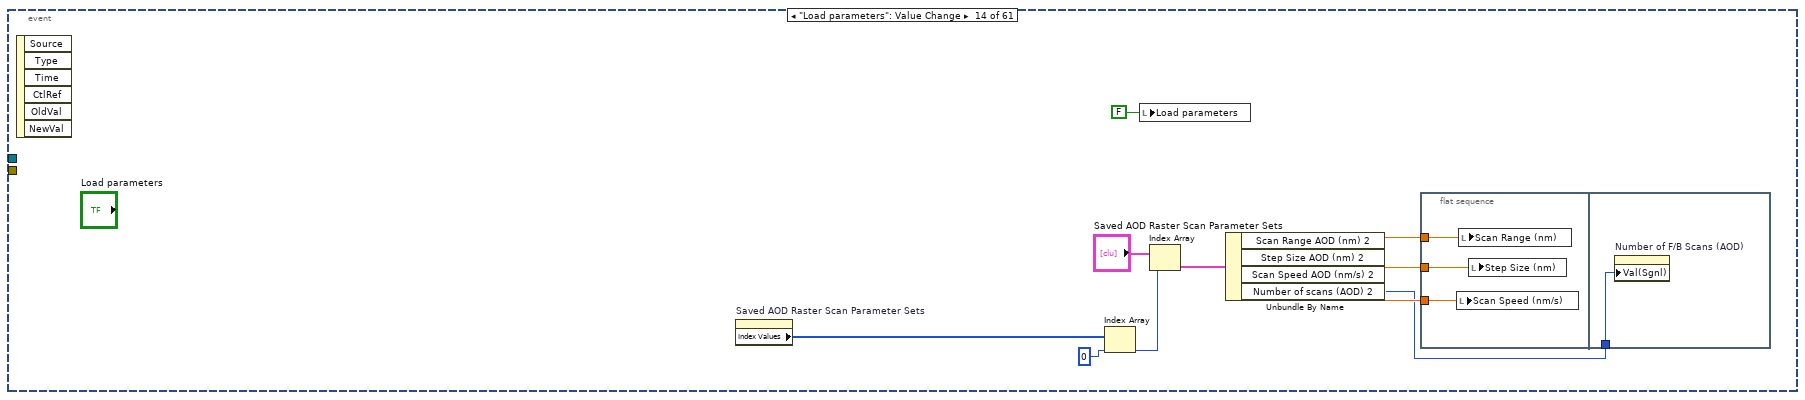
[diagram p18: hidden frame]
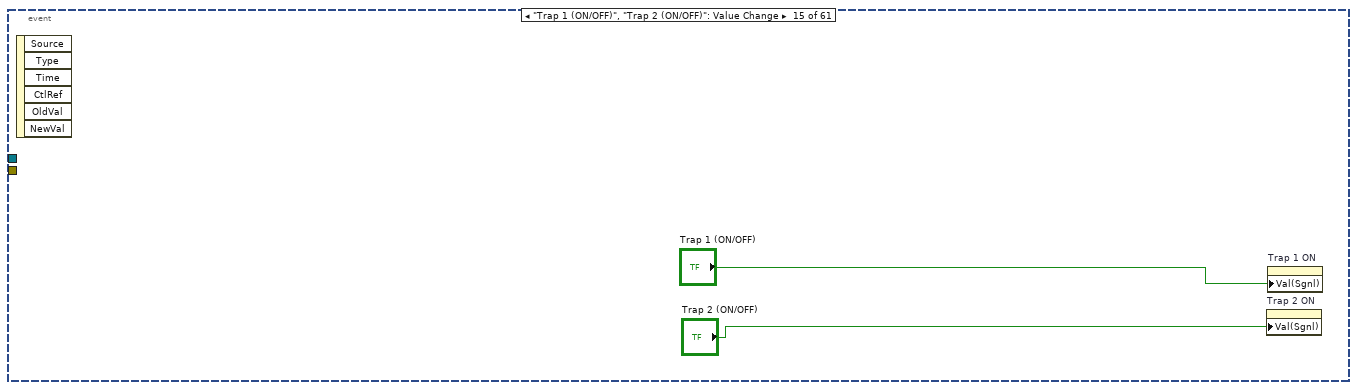
[diagram p19: hidden frame]
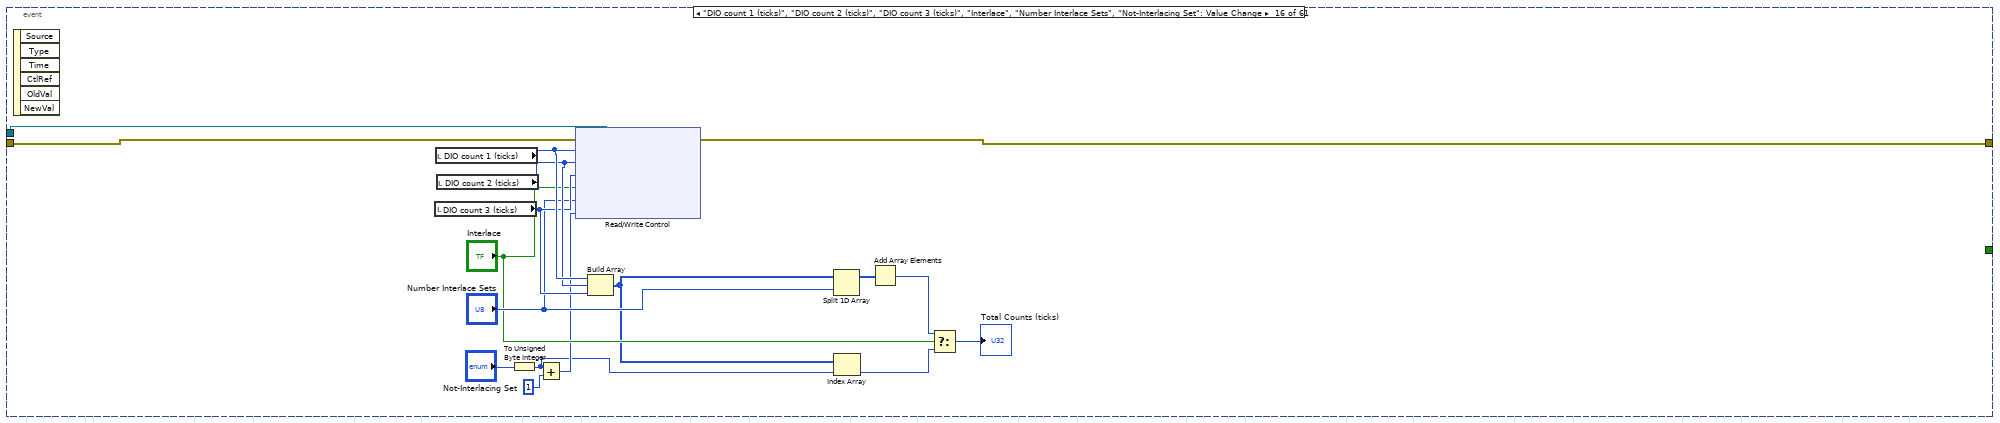
[diagram p20: hidden frame]
diagram:
  n1 = node-c288() -> (w2:T11)  [unwired: 4 in]
  n2 = timed-loop "Control parameters (event loop)" {
    tunnel: _ -> [w5]
    shift-right: [w4] -> _
    shift-left: _ -> [w3]
    timing: w2 -> [_]
    timing-out: [_] -> w1
    stop <- _ stop-if-true
    n3 = node-c288() -> ()  [unwired: 1 in, 1 out]
    n4 = event shown="[41]" {
      selector: _ -> [_ _ _ _ _ _ _ _ _ _ _ _ _ _ _ _ _ _ _ _ _ _ _ _ _ _ _ _ _ _ _ _ _ _ _ _ _ _ _ _ _ _ _ _ _ _ _ _ _ _ _ _ _ _ _ _ _ _ _ _ _]
      dyn-events: _ -> [_ _ _ _ _ _ _ _ _ _ _ _ _ _ _ _ _ _ _ _ _ _ _ _ _ _ _ _ _ _ _ _ _ _ _ _ _ _ _ _ _ _ _ _ _ _ _ _ _ _ _ _ _ _ _ _ _ _ _ _ _]
      timeout: _ -> [_ _ _ _ _ _ _ _ _ _ _ _ _ _ _ _ _ _ _ _ _ _ _ _ _ _ _ _ _ _ _ _ _ _ _ _ _ _ _ _ _ _ _ _ _ _ _ _ _ _ _ _ _ _ _ _ _ _ _ _ _]
      tunnel: w5 -> [w45 _ _ _ w82 _ w100 w104 _ _ _ _ w164 _ _ w208 w214 w218 w223 w259 w274 w279 w295 w306 w317 w328 w339 w350 w368 w374 w461 _ w471 w506 _ w566 w570 w581 w586 w607 _ w615 _ _ _ _ _ w749 _ w766 w781 w806 w809 w810 w862 _ w879 w881 _ _ _]
      tunnel: [w44 _ _ _ w72 _ _ w103 _ _ w130 _ w144 _ _ w207 w210 w217 w220 w258 w272 w278 w289 w300 w311 w322 w333 w344 w366 w373 w459 _ w469 w504 _ w564 w568 w571 w584 w605 _ w613 _ _ _ _ _ w747 _ _ _ _ _ _ _ _ _ _ _ _ _] -> w4
      tunnel: w3 -> [w43 _ _ _ w81 _ _ w102 _ _ w130 _ w163 _ _ w206 w209 w216 w219 w257 w273 w277 w294 w305 w316 w327 w338 w349 w367 w372 w460 _ w470 w505 _ w565 w569 w580 w585 w606 _ w614 _ _ _ _ _ w748 _ w765 w780 w805 w808 w811 w861 _ w878 _ _ _ _]
      tunnel: [_ _ _ _ _ _ _ _ _ _ w129 _ _ _ _ _ _ _ _ _ _ _ _ _ _ _ _ _ _ _ _ _ _ _ _ _ _ _ _ _ _ _ _ _ _ _ _ _ _ _ _ _ _ _ _ _ _ _ _ _ _] -> _
      tunnel: [_ _ _ _ _ _ _ _ "Round T1 X" _ _ _ _ _ _ _ _ _ _ _ _ _ _ _ _ _ _ _ _ _ _ _ _ _ _ _ _ _ _ _ _ _ _ _ _ _ _ _ _ _ _ _ _ _ _ _ _ _ _ _ _] -> _
      tunnel: [_ _ _ "Adjust Scale\nto Mean" _ _ _ _ _ _ _ _ _ _ _ _ _ _ _ _ _ _ _ _ _ _ _ _ _ _ _ _ _ _ _ _ _ _ _ _ _ _ _ _ _ _ _ _ _ _ _ _ _ _ "Set SP to Reading" _ _ _ _ _ _] -> _
      tunnel: [_ _ _ _ _ _ _ _ _ "Round T2 X" _ "Delayed Interlace Start" _ _ _ _ _ _ _ _ _ _ _ _ _ _ _ _ _ _ _ _ _ _ _ _ _ _ _ _ _ _ _ _ _ _ _ _ _ _ _ _ _ _ _ _ _ _ _ _ _] -> _
      event "AI Count (ticks)", "Sets to FIFO (Traps)", "# Samples/channel", "N sets to save": Value Change {
        # "So that if 'Save ave N' is updated, the AOD scanning code updates too."
        n5 = event-data() -> ()  [unwired: 6 out]
        n6 = local read "AI Count (ticks)"() -> (w27:u32)
        n7 = Unbundle By Name("Sets to FIFO (Traps)") -> ("Set 1"=w10:bool, "Set 2"=w9:bool, "Set 3"=w8:bool)
        n8 = Boolean To (0,1)(Boolean="Sets to FIFO (Traps)") -> (0, 1=w36:cluster{"Set 1":i16, "Set 2":i16, "Set 3":i16})
        n9 = xnode "Read/Write Control"("FPGA VI Reference In"=w45, "error in"=w43, "ai count"=w27, "Set 1"=w10, "Set 2"=w9, "Set 3"=w8, "N of AI1 Int Acq Sets"="N Acq Sets (Traps + Fl.)") -> ("error out"=w44:errorcluster)  [unwired: 1 out]
        n10 = Cluster To Array(cluster=w36) -> (array=w35:i16[])
        n11 = To Unsigned Long Integer(number=w35) -> (unsigned 32bit integer=w16:u32[])
        n12 = local read "Scan steps (AOD)"() -> (w37:u64)
        n13 = Multiply(x=w27, y="N Acq Sets (Traps + Fl.)") -> (x*y=w25:u32)
        n14 = Divide(x=40000000.0, y=w27) -> (x/y=w19:dbl)
        "AI rate (Hz)" <- w19
        "Ave. Rate (Hz)" <- w19
        n15 = Add Array Elements(numeric array=w16) -> (sum=w28:u32)
        "Trap Sets" <- w28
        n16 = Reciprocal(x=w19) -> (1/x=→"Ave. Period (s)":dbl)
        n17 = property on="Scan steps (AOD)" class="DigNum (strict)"("Val(Sgnl)"=w37) -> ()  [unwired: 2 in, 2 out]
        n18 = Divide(x=w19, y="N Acq Sets (Traps + Fl.)") -> (x/y=w40:dbl)
        "Data Rate (Hz)" <- w40
        n19 = Reciprocal(x=w40) -> (1/x=→"Data Period (s)":dbl)
        n20 = local read item#-1() -> ()  [unwired: 1 out]
        n21 = Divide(x=w40) -> (x/y=w39:dbl)  [unwired: 1 in]
        "Save Data Rate (Hz)" <- w39
        n22 = Reciprocal(x=w39) -> (1/x=→"Save Data Period (s)":dbl)
        n23 = Multiply(x=w25, y="# Samples/trap") -> (x*y=w23:u32)
        "Counts/DMA" <- w23
        n24 = property on="Property Node" class="DigNum (strict)"("Maximum"="# Samples/trap") -> ()  [unwired: 2 in, 2 out]
        n25 = Multiply(x=w28, y="# Samples/trap") -> (x*y=w17:u32)
        "# Samples/channel" <- w17
        n26 = Multiply(x=w17, y=u32 8) -> (x*y=→"Trap AI Elements/DMA read":u32)
        n27 = local read "APD Int. Count"() -> (w24:u32)
        n28 = Multiply(x=w17, y=u32 3) -> (x*y=→"Trap Pos Elements/DMA read":u32)
        n29 = Divide(x=w23, y=w24) -> (x/y=w14:dbl)
        "APD Samples/FIFO Acq." <- w14
        n30 = Divide(x=w23, y=40000000.0) -> (x/y=w21:dbl)
        "DMA Update Period (s)" <- w21
        n31 = property on="Property Node" class="DigNum (strict)"("Maximum"=w14) -> ()  [unwired: 2 in, 2 out]
        n32 = Multiply(x=2.0, y=w14) -> (x*y=→"APD Elements/DMA read":dbl)
        n33 = local read "N sets to save"() -> (w33:u32)
        n34 = Multiply(x=w21, y=w33) -> (x*y=→"Total Time (s)":dbl)
        "FPGA Averaging" <- FALSE ("FPGA Averaging")
      }
      event "Rescale on Mean": Value Change {
        n35 = event-data() -> ()  [unwired: 7 out]
        n36 = And(x=FALSE, y="Rescale on Mean") -> (x .and. y?=w47:bool)
        n37 = local write "Rescale on Mean"(w47) -> ()
        n38 = local read "Bead Mean (nm)"() -> (w52:dbl)
        n39 = Add(x="Amplitude (nm)", y=w52) -> (x+y=w50:dbl)
        n40 = Subtract(x=w52, y="Amplitude (nm)") -> (x-y=w49:dbl)
        n41 = property on="Property Node" class="WFChart (strict)"("YScale.Minimum"=w49) -> ()  [unwired: 2 in, 2 out]
        n42 = property on="Property Node" class="WFChart (strict)"("YScale.Maximum"=w50) -> ()  [unwired: 2 in, 2 out]
      }
      event #2 (no event record) {
        n43 = event-data() -> ()  [unwired: 7 out]
        n44 = local read "AI labels"() -> (w53:string[])
        n45 = property on="Property Node" class="Ring (strict)"("Strings []"=w53) -> ()  [unwired: 2 in, 2 out]
        n46 = Build Array (concatenate)(w53, "none") -> (w54:string[])
        n47 = property on="Property Node" class="Ring (strict)"("Strings []"=w54) -> ()  [unwired: 2 in, 2 out]
        n48 = property on="Property Node" class="Ring (strict)"("Strings []"=w54) -> ()  [unwired: 2 in, 2 out]
        n49 = property on="Property Node" class="Ring (strict)"("Strings []"=w54) -> ()  [unwired: 2 in, 2 out]
        n50 = property on="Property Node" class="Ring (strict)"("Strings []"=w54) -> ()  [unwired: 2 in, 2 out]
        n51 = Bundle("APD 1", "APD 2") -> (w57:cluster{string, string})  [unwired: 1 out]
        n52 = Cluster To Array(cluster=w57) -> (array=w55:string[])
        n53 = Build Array (concatenate)(w55, w54) -> (w59:string[])
        n54 = Array Size(array=w59) -> (size(s)=w60:i32)
        n55 = property on="Property Node" class="LstBox (strict)"("Item Names"=w59) -> ()  [unwired: 2 in, 2 out]
        n56 = property on="Property Node" class="LstBox (strict)"("Number of Rows"=w60) -> ()  [unwired: 2 in, 2 out]
        n57 = property on="Property Node" class="WFChart (strict)"("LegNumRows"=w60) -> ()  [unwired: 2 in, 2 out]
      }
      event "Adjust Scale\nto Mean": Value Change {
        n58 = event-data() -> ()  [unwired: 7 out]
        n59 = local read "APD 1 Rate (Hz)"() -> (w69:dbl)
        n60 = Multiply(x=1000.0, y="Above (kHz)") -> (x*y=w67:dbl)
        n61 = Multiply(x=1000.0, y="Below (kHz)") -> (x*y=w65:dbl)
        n62 = Add(x=w67, y=w69) -> (x+y=w62:dbl)
        n63 = Subtract(x=w69, y=w65) -> (x-y=w63:dbl)
        n64 = property on="Property Node" class="WFChart (strict)"("YScale.Minimum"=w63) -> ()  [unwired: 2 in, 2 out]
        n65 = property on="Property Node" class="WFChart (strict)"("YScale.Maximum"=w62) -> ()  [unwired: 2 in, 2 out]
      }
      event "Phase adj. (AI1)", "+ phase (AI1)", "- phase (AI1)": Value Change {
        n66 = event-data() -> ()  [unwired: 7 out]
        n67 = Negate(x="Phase adj. (AI1)") -> (-x=w79:i16)
        n68 = Select(t=w79, s="- phase (AI1)", f="Phase adj. (AI1)") -> (s? t:f=w78:i16)
        n69 = xnode "Read/Write Control"("FPGA VI Reference In"=w82, "error in"=w81, "Phase count adjustment"=w78) -> ("FPGA VI Reference Out"=w77:T17, "error out"=w76:errorcluster)
        n70 = Or(x="- phase (AI1)", y="+ phase (AI1)") -> (x .or. y?=w73:bool)
        n71 = xnode "Read/Write Control"("FPGA VI Reference In"=w77, "error in"=w76, "+ phase"=w73) -> ("error out"=w72:errorcluster)  [unwired: 1 out]
      }
      event #5 (no event record) {
        w85 = u32 9868950 ("Color Box")
        n72 = event-data() -> ("Row"=w87)  [unwired: 9 out]
        n73 = property on="Property Node" class="WFChart (strict)"("Active Plot"=w87) -> (error out=w98:errorcluster)  [unwired: 2 in, 1 out]
        n74 = property on="Property Node" class="WFChart (strict)" props=["Plot", "Visible?", "Plot", "Plot Color"](error in=w98) -> (error out=w97:errorcluster, "Plot.Visible?"=w96:bool)  [unwired: 1 in, 2 out]
        n75 = Select(t=FALSE ("Plot.Visible"), s=w96, f=TRUE ("Plot.Visible")) -> (s? t:f=w91:bool)
        n76 = property on="Property Node" class="WFChart (strict)"(error in=w97, "Plot.Visible?"=w91) -> (error out=w93:errorcluster)  [unwired: 1 in, 1 out]
        n77 = property on="Property Node" class="WFChart (strict)"(error in=w93) -> (error out=w88:errorcluster, "Plot.Plot Color"=w92:u32)  [unwired: 1 in, 1 out]
        n78 = property on="Property Node" class="LstBox (strict)"(error in=w88, "Active Row"=w87) -> (error out=w86:errorcluster)  [unwired: 1 in, 1 out]
        n79 = Select(t=w92, s=w91, f=u32 0) -> (s? t:f=w89:u32)
        n80 = property on="Property Node" class="LstBox (strict)"(error in=w86, "CellFontColor"=w89, "SelColor"=w85, "CellBG"=w85, "CellFontSize"=u32 20 ("Active Row:Cell Font:Size"), "CellFontBold"=TRUE ("Active Row:Cell Font:Bold")) -> ()  [unwired: 1 in, 2 out]
      }
      event "Dynamic Force FB": Value Change {
        n81 = event-data() -> ()  [unwired: 7 out]
        n82 = xnode "Read/Write Control"("FPGA VI Reference In"=w100, "Dynamic Force FB (Ronen)"="Dynamic Force FB") -> ()  [unwired: 1 in, 2 out]
      }
      event #7 (no event record) {
        # "anytime one of the frequencies is changed, write it to the RF board UNLESS Set 2 is being oscillated. The oscillation\nscript writes the frequencies to the RF board."
        n83 = event-data() -> ()  [unwired: 7 out]
        n84 = Equal?() -> (x = y?=w101:bool)  [unwired: 2 in]
        n85 = case shown="False" "Oscillate Set 2" {
          tunnel: w104 -> [w117 _]
          tunnel: [w116 w125] -> w103
          tunnel: w102 -> [w115 w125]
          tunnel: w101 -> [w107 _]
          frame False {
            n86 = case shown="False" "Symmetric manual \ntrap motion" {
              tunnel: ["T2 for asymmetric\n(MHz)" w124] -> w108
              tunnel: [w119 w121] -> _
              frame False {
                n87 = Subtract(x="T2 for asymmetric\n(MHz)") -> (x-y=w119:dbl)  [unwired: 1 in]
              }
              frame True {
                n88 = Divide(y=2) -> (x/y=w122:dbl)  [unwired: 1 in]
                n89 = Subtract(x="Middle freq for \nsymmetric (MHz)", y=w122) -> (x-y=w121:dbl)
                n90 = Add(x="Middle freq for \nsymmetric (MHz)", y=w122) -> (x+y=w124:dbl)
              }
            }
            n91 = local read item#-1() -> (w109)
            n92 = local read item#-1() -> ()  [unwired: 1 in]
            n93 = Select(t=w108, s=w107, f=w109) -> ()  [unwired: 1 out]
            n94 = local read item#-1() -> ()  [unwired: 1 out]
            n95 = local read item#-1() -> ()  [unwired: 1 out]
            n96 = local read item#-1() -> ()  [unwired: 1 out]
            n97 = local read item#-1() -> ()  [unwired: 1 in]
            n98 = local read item#-1() -> ()  [unwired: 1 out]
            n99 = local read item#-1() -> ()  [unwired: 1 out]
            n100 = local read item#-1() -> ()  [unwired: 1 out]
            n101 = call "set RF board frequency - interlace.vi"("error in"=w115, "FPGA VI Reference In"=w117) -> ("error out"=w116:errorcluster)  [unwired: 8 in, 1 out]
            n102 = Subtract() -> (x-y=w113:dbl)  [unwired: 2 in]
            n103 = Subtract() -> (x-y=w114:dbl)  [unwired: 2 in]
            n104 = Square(x=w113) -> (x^2=w111:dbl)
            n105 = Square(x=w114) -> (x^2=w112:dbl)
            n106 = Add(x=w112, y=w111) -> (x+y=w110:dbl)
            n107 = Square Root(x=w110) -> ()  [unwired: 1 out]
            n108 = local read item#-1() -> ()  [unwired: 1 in]
            n109 = property on="Initial delta (MHz)" class="DigNum (strict)" props=["Val(Sgnl)"]() -> ()  [unwired: 3 in, 2 out]
          }
          frame True {
          }
        }
      }
      event "Round T1 X": Value Change {
        n110 = event-data() -> ()  [unwired: 7 out]
        n111 = local read item#-1() -> ()  [unwired: 1 out]
        n112 = Round To Nearest() -> ()  [unwired: 1 in, 1 out]
      }
      event "Round T2 X": Value Change {
        n113 = event-data() -> ()  [unwired: 7 out]
        n114 = local read item#-1() -> ()  [unwired: 1 out]
        n115 = Round To Nearest() -> ()  [unwired: 1 in, 1 out]
      }
      event #10 (no event record) {
        n116 = event-data() -> ()  [unwired: 7 out]
        n117 = call "hamilton_controller.vi"("action"=T14."DISCONNECT") -> ()  [unwired: 10 in, 1 out]
        n118 = local read item#-1() -> (w129)
      }
      event "Delayed Interlace Start": Value Change {
        n119 = event-data() -> ()  [unwired: 7 out]
        n120 = flat-sequence {
          frame #0 {
            n121 = Multiply(x="Delay to Interlace (s)", y=1000.0) -> (x*y=w132:dbl)
            n122 = Wait (ms)(milliseconds to wait=w132) -> ()  [unwired: 1 out]
          }
          frame #1 {
            (unwired) enum32{"Laser ON", "Laser OFF", "Interlace"}."Interlace" ("Value (Signaling)")
          }
        }
      }
      event "BD 1 Amplitude 1 (%)", "BD 1 Amplitude 2 (%)", "BD 1 Amplitude 3 (%)", "BD 2 Amplitude 1 (%)", "BD 2 Amplitude 2 (%)", "BD 2 Amplitude 3 (%)", "Trap 1 ON", "Trap 2 ON", "Trap 3 ON", "Feedback On/Off", "All FB On/Off": Value Change {
        w155 = i16 1 ("f")
        n123 = event-data() -> ()  [unwired: 7 out]
        n124 = local write "Trap 1 (ON/OFF)"("Trap 1 ON") -> ()
        n125 = local write "Trap 2 (ON/OFF)"("Trap 2 ON") -> ()
        n126 = Boolean To (0,1)(Boolean="Trap 3 ON") -> (0, 1=w156:i16)
        n127 = Boolean To (0,1)(Boolean="Trap 1 ON") -> (0, 1=w157:i16)
        n128 = Boolean To (0,1)(Boolean="Trap 2 ON") -> (0, 1=w158:i16)
        n129 = Select(t=w158, s="Trap ON/OFF X or Y Amp?", f=w155) -> (s? t:f=w153:i16)
        n130 = Select(t=w157, s="Trap ON/OFF X or Y Amp?", f=w155) -> (s? t:f=w154:i16)
        n131 = Select(t=w156, s="Trap ON/OFF X or Y Amp?", f=w155) -> (s? t:f=w152:i16)
        n132 = Select(t=w155, s="Trap ON/OFF X or Y Amp?", f=w158) -> (s? t:f=w150:i16)
        n133 = Select(t=w155, s="Trap ON/OFF X or Y Amp?", f=w157) -> (s? t:f=w151:i16)
        n134 = Select(t=w155, s="Trap ON/OFF X or Y Amp?", f=w156) -> (s? t:f=w149:i16)
        n135 = And(x="All FB On/Off", y="Feedback On/Off") -> (x .and. y?=w147:cluster{"Set 1":bool, "Set 2":bool})
        n136 = local read "BD 1 Amplitude 1 (%)"() -> (w167:dbl)
        n137 = local read "BD 1 Amplitude 2 (%)"() -> (w166:dbl)
        n138 = local read "BD 1 Amplitude 3 (%)"() -> (w165:dbl)
        n139 = Unbundle By Name(w147) -> ("Set 1"=w143:bool, "Set 2"=w140:bool)
        n140 = local read "Y RF Amplitude Limits (%)"() -> (w136:T5)
        n141 = local read "X RF Amplitude Limits (%)"() -> (w137:T5)
        n142 = local read "BD 2 Amplitude 1 (%)"() -> (w168:dbl)
        n143 = local read "BD 2 Amplitude 2 (%)"() -> (w169:dbl)
        n144 = local read "BD 2 Amplitude 3 (%)"() -> (w170:dbl)
        n145 = And(x="Trap 2 ON", y=w140) -> (x .and. y?=w138:bool)
        n146 = And(x="Trap 1 ON", y=w143) -> (x .and. y?=w141:bool)
        n147 = Multiply(x=w154, y=w167) -> (x*y=w162:dbl)
        n148 = Multiply(x=w166, y=w153) -> (x*y=w160:dbl)
        n149 = Multiply(x=w165, y=w152) -> (x*y=w161:dbl)
        n150 = Multiply(x=w168, y=w151) -> (x*y=w171:dbl)
        n151 = Multiply(x=w169, y=w150) -> (x*y=w172:dbl)
        n152 = Multiply(x=w170, y=w149) -> (x*y=w173:dbl)
        n153 = call "set RF board amplitude - interlace.vi"("Board 2 Amplitude Limits"=w136, "Board 1 Amplitude Limits"=w137, "error in"=w163, "FPGA VI Reference In"=w164, "Board 2 Amplitude 3 (%)"=w173, "Board 1 Amplitude 3 (%)"=w161, "Board 2 Amplitude 2 (%)"=w172, "Board 2 Amplitude 1 (%)"=w171, "Board 1 Amplitude 2 (%)"=w160, "Board 1 Amplitude 1 (%)"=w162) -> ("error out"=w145:errorcluster, "FPGA VI Reference Out"=w146:T17)
        n154 = xnode "Read/Write Control"("FPGA VI Reference In"=w146, "error in"=w145, "FB On/Off Set 1"=w141, "FB On/Off Set 2"=w138) -> ("error out"=w144:errorcluster)  [unwired: 1 out]
        n155 = case shown="True" "All FB On/Off" {
          frame False {
          }
          frame True {
            n156 = local write "Feedback overload"(FALSE) -> ()
          }
        }
      }
      event "Load parameters": Value Change {
        n157 = event-data() -> ()  [unwired: 7 out]
        n158 = property on="Saved AOD Raster Scan Parameter Sets" class="Arr (strict)"() -> ("Index Values"=w185:u32[])  [unwired: 2 in, 2 out]
        n159 = Index Array(array=w185, index=0) -> (element=w182:u32)
        n160 = local write "Load parameters"(FALSE ("Load parameters")) -> ()
        n161 = Index Array(array="Saved AOD Raster Scan Parameter Sets", index=w182) -> (element=w181:T18)
        n162 = Unbundle By Name(w181) -> ("Scan Range AOD (nm) 2"=w180:dbl, "Step Size AOD (nm) 2"=w179:dbl, "Scan Speed AOD (nm/s) 2"=w178:dbl, "Number of scans (AOD) 2"=w177:u16)
        n163 = flat-sequence {
          tunnel: w180 -> [w188]
          tunnel: w179 -> [w187]
          tunnel: w178 -> [w186]
          tunnel: w177 -> [w189]
          frame #0 {
            n164 = local write "Scan Speed (nm/s)"(w186) -> ()
            n165 = local write "Scan Range (nm)"(w188) -> ()
            n166 = local write "Step Size (nm)"(w187) -> ()
          }
          frame #1 {
            n167 = property on="Number of F/B Scans (AOD)" class="DigNum (strict)"("Val(Sgnl)"=w189) -> ()  [unwired: 2 in, 2 out]
          }
        }
      }
      event "Trap 1 (ON/OFF)", "Trap 2 (ON/OFF)": Value Change {
        n168 = event-data() -> ()  [unwired: 7 out]
        n169 = property on="Trap 2 ON" class="Bool (strict)"("Val(Sgnl)"="Trap 2 (ON/OFF)") -> ()  [unwired: 2 in, 2 out]
        n170 = property on="Trap 1 ON" class="Bool (strict)"("Val(Sgnl)"="Trap 1 (ON/OFF)") -> ()  [unwired: 2 in, 2 out]
      }
      event "DIO count 1 (ticks)", "DIO count 2 (ticks)", "DIO count 3 (ticks)", "Interlace", "Number Interlace Sets", "Not-Interlacing Set": Value Change {
        n171 = event-data() -> ()  [unwired: 7 out]
        n172 = local read "DIO count 3 (ticks)"() -> (w202:u32)
        n173 = local read "DIO count 1 (ticks)"() -> (w204:u32)
        n174 = local read "DIO count 2 (ticks)"() -> (w203:u32)
        n175 = To Unsigned Byte Integer(number="Not-Interlacing Set") -> (unsigned 8bit integer=w193:u8)
        n176 = Add(x=w193, y=u8 1) -> (x+y=w197:u8)
        n177 = xnode "Read/Write Control"("FPGA VI Reference In"=w208, "error in"=w206, "DIO count 1 (ticks)"=w204, "DIO count 2 (ticks)"=w203, "DIO count 3 (ticks)"=w202, "Interlace ON/OFF"="Interlace", "Number Interlace Cycles"="Number Interlace Sets", "Interlace Off Parameters"=w197) -> ("error out"=w207:errorcluster)  [unwired: 1 out]
        n178 = Build Array(w204, w203, w202) -> (w195:u32[])
        n179 = Split 1D Array(array=w195, index="Number Interlace Sets") -> (first subarray=w205:u32[])  [unwired: 1 out]
        n180 = Index Array(array=w195, index=w193) -> (element=w194:u32)
        n181 = Add Array Elements(numeric array=w205) -> (sum=w199:u32)
        n182 = Select(t=w199, s="Interlace", f=w194) -> (s? t:f=→"Total Counts (ticks)":u32)
      }
      event "Reset Feedback": Value Change {
        n183 = event-data() -> ()  [unwired: 7 out]
        n184 = Unbundle By Name("Reset Feedback") -> ("Set 1"=w212:bool, "Set 2"=w211:bool)
        n185 = xnode "Read/Write Control"("FPGA VI Reference In"=w214, "error in"=w209, "FB Reset Set 1"=w212, "FB Reset Set 2"=w211) -> ("error out"=w210:errorcluster)  [unwired: 1 out]
      }
      event "PID gains": Value Change {
        n186 = event-data() -> ()  [unwired: 7 out]
        n187 = local read "PID gains"() -> (w215:T4)
        n188 = xnode "Read/Write Control"("FPGA VI Reference In"=w218, "error in"=w216, "FB Gains"=w215) -> ("error out"=w217:errorcluster)  [unwired: 1 out]
      }
      event "AI2 to Setpoint", "Trap Intensity\nSetpoints (V)": Value Change {
        n189 = event-data() -> ()  [unwired: 7 out]
        n190 = xnode "Read/Write Control"("FPGA VI Reference In"=w223, "error in"=w219) -> ("FPGA VI Reference Out"=w222:T17, "error out"=w221:errorcluster, "AI2 Y Sum Set 1"=w230:i16, "AI2 Y Sum Set 2"=w229:i16)
        n191 = Cluster To Array(cluster="AI2 to Setpoint") -> (array=w233:bool[])
        n192 = local read "AI2 (V)"() -> (w231:cluster{"Set 1":dbl, "Set 2":dbl})
        n193 = Or Array Elements(Boolean array=w233) -> (logical OR=w234:bool)
        n194 = Bundle By Name(cluster=w231, "Set 1"=w230, "Set 2"=w229) -> (w228:cluster{"Set 1":dbl, "Set 2":dbl})
        n195 = Divide(x=w228, y=3276.7) -> (x/y=w227:cluster{"Set 1":dbl, "Set 2":dbl})
        "AI2 (V)" <- w227
        n196 = case shown="False" w234 {
          tunnel: [w237 w254] -> w226
          tunnel: "AI2 to Setpoint" -> [_ w250]
          tunnel: "Trap Intensity\nSetpoints (V)" -> [w238 w253]
          tunnel: w227 -> [_ w247]
          frame False {
            n197 = Multiply(x=3276.7, y=w238) -> (x*y=w239:cluster{"Set 1":dbl, "Set 2":dbl})
            n198 = To Word Integer(number=w239) -> (16bit integer=w237:cluster{"Set 1":i16, "Set 2":i16})
          }
          frame True {
            n199 = Unbundle By Name(w247) -> ("Set 1"=w246:dbl, "Set 2"=w245:dbl)
            n200 = Unbundle By Name(w253) -> ("Set 1"=w252:dbl, "Set 2"=w251:dbl)
            n201 = Unbundle By Name(w250) -> ("Set 1"=w249:bool, "Set 2"=w248:bool)
            n202 = Select(t=w246, s=w249, f=w252) -> (s? t:f=w244:dbl)
            n203 = Select(t=w245, s=w248, f=w251) -> (s? t:f=w243:dbl)
            n204 = Bundle By Name(cluster=w253, "Set 1"=w244, "Set 2"=w243) -> (w241:cluster{"Set 1":dbl, "Set 2":dbl})
            n205 = local write "Trap Intensity\nSetpoints (V)"(w241) -> ()
            n206 = Multiply(x=3276.7, y=w241) -> (x*y=w242:cluster{"Set 1":dbl, "Set 2":dbl})
            n207 = To Word Integer(number=w242) -> (16bit integer=w254:cluster{"Set 1":i16, "Set 2":i16})
          }
        }
        n208 = Unbundle By Name(w226) -> ("Set 1"=w225:i16, "Set 2"=w224:i16)
        n209 = xnode "Read/Write Control"("FPGA VI Reference In"=w222, "error in"=w221, "FB Setpoint Set 1"=w225, "FB Setpoint Set 2"=w224) -> ("error out"=w220:errorcluster)  [unwired: 1 out]
      }
      event "Invert GI": Value Change {
        n210 = event-data() -> ()  [unwired: 7 out]
        n211 = xnode "Read/Write Control"("FPGA VI Reference In"=w259, "error in"=w257, "Invert GI"="Invert GI", "Invert GI 2"="Invert GI") -> ("error out"=w258:errorcluster)  [unwired: 1 out]
      }
      event "Green FB Setpoint (mV)", "Green FB Gains", "Current When FB OFF (%)", "Green int current ON count adj": Value Change {
        n212 = event-data() -> ()  [unwired: 7 out]
        n213 = local read "Green FB Setpoint (mV)"() -> (w264:dbl)
        n214 = local read "Current When FB OFF (%)"() -> (w267:dbl)
        n215 = Multiply(x=w264, y=3.2767) -> (x*y=w263:dbl)
        n216 = Multiply(x=w267, y=655.35) -> (x*y=w268:dbl)
        n217 = To Unsigned Word Integer(number=w268) -> (unsigned 16bit integer=w266:u16)
        n218 = local read "Green int current ON count adj"() -> (w271:u32)
        n219 = local read "Green FB Gains"() -> (w270:T4)
        n220 = local read item#-1() -> ()  [unwired: 1 out]
        n221 = local read item#-1() -> ()  [unwired: 1 out]
        n222 = local read item#-1() -> ()  [unwired: 1 out]
        n223 = Equal?(y=enum32{"Laser ON", "Laser OFF", "Interlace"}."Interlace") -> (x = y?=w260:bool)  [unwired: 1 in]
        n224 = Compound Arithmetic op=AND(w260) -> (w262:bool)  [unwired: 2 in]
        n225 = xnode "Read/Write Control"("FPGA VI Reference In"=w274, "error in"=w273, "Green FB Setpoint"=w263, "Green FB On/Off"=w262, "Current Out"=w266, "Green int current ON count adj"=w271, "Green FB Gains"=w270) -> ("error out"=w272:errorcluster)  [unwired: 1 out]
      }
      event #21 (no event record) {
        n226 = event-data() -> ()  [unwired: 7 out]
        n227 = case shown="True" {
          selector: _ -> [_ _]
          tunnel: [enum32{"Laser ON", "Laser OFF", "Interlace"}."Laser OFF" ("Green laser mode") _] -> w276
          tunnel: [FALSE w282] -> w275
          frame False {
          }
          frame True {
            n228 = local read item#-1() -> ()  [unwired: 1 out]
            n229 = Equal?(y=enum32{"Laser ON", "Laser OFF", "Interlace"}."Interlace") -> (x = y?=w283:bool)  [unwired: 1 in]
            n230 = And(x=w283) -> (x .and. y?=w282:bool)  [unwired: 1 in]
          }
        }
        n231 = xnode "Read/Write Control"("FPGA VI Reference In"=w279, "error in"=w277, "Operating Mode"=w276, "Operating Mode 2"=w276, "Green FB On/Off"=w275) -> ("error out"=w278:errorcluster)  [unwired: 1 out]
      }
      event "- phase (APD 1 Gate)", "+ phase (APD 1 Gate)": Value Change {
        n232 = event-data() -> ()  [unwired: 7 out]
        n233 = local read "Phase Adj. (APD 1 Gate)"() -> (w285:i16)
        n234 = Negate(x=w285) -> (-x=w293:i16)
        n235 = Select(t=w293, s="- phase (APD 1 Gate)", f=w285) -> (s? t:f=w292:i16)
        n236 = Or(x="- phase (APD 1 Gate)", y="+ phase (APD 1 Gate)") -> (x .or. y?=w288:bool)
        n237 = xnode "Read/Write Control"("FPGA VI Reference In"=w295, "error in"=w294, "Phase count adjustment (APD 1 Gate)"=w292) -> ("FPGA VI Reference Out"=w290:T17, "error out"=w291:errorcluster)
        n238 = xnode "Read/Write Control"("FPGA VI Reference In"=w290, "error in"=w291, "+ phase (APD 1 Gate)"=w288) -> ("error out"=w289:errorcluster)  [unwired: 1 out]
      }
      event "+ phase (APD 2 Gate)", "- phase (APD 2 Gate)": Value Change {
        n239 = event-data() -> ()  [unwired: 7 out]
        n240 = local read "Phase Adj. (APD 2 Gate)"() -> (w296:i16)
        n241 = Negate(x=w296) -> (-x=w304:i16)
        n242 = Select(t=w304, s="- phase (APD 2 Gate)", f=w296) -> (s? t:f=w303:i16)
        n243 = Or(x="- phase (APD 2 Gate)", y="+ phase (APD 2 Gate)") -> (x .or. y?=w299:bool)
        n244 = xnode "Read/Write Control"("FPGA VI Reference In"=w306, "error in"=w305, "Phase count adjustment (APD 2 Gate)"=w303) -> ("FPGA VI Reference Out"=w301:T17, "error out"=w302:errorcluster)
        n245 = xnode "Read/Write Control"("FPGA VI Reference In"=w301, "error in"=w302, "+ phase (APD 2 Gate)"=w299) -> ("error out"=w300:errorcluster)  [unwired: 1 out]
      }
      event "Phase Adj. (APD Acq)", "+ phase (APD Acq)", "- phase (APD Acq)": Value Change {
        n246 = event-data() -> ()  [unwired: 7 out]
        n247 = local read "Phase Adj. (APD Acq)"() -> (w309:i16)
        n248 = Negate(x=w309) -> (-x=w315:i16)
        n249 = Select(t=w315, s="+ phase (APD Acq)", f=w309) -> (s? t:f=w314:i16)
        n250 = Or(x="+ phase (APD Acq)", y="- phase (APD Acq)") -> (x .or. y?=w310:bool)
        n251 = xnode "Read/Write Control"("FPGA VI Reference In"=w317, "error in"=w316, "Phase Count Adjustment (APD Acq)"=w314) -> ("FPGA VI Reference Out"=w312:T17, "error out"=w313:errorcluster)
        n252 = xnode "Read/Write Control"("FPGA VI Reference In"=w312, "error in"=w313, "+ phase (APD Acq)"=w310) -> ("error out"=w311:errorcluster)  [unwired: 1 out]
      }
      event "Phase adj. (GI)", "+ phase (GI)", "- phase (GI)": Value Change {
        n253 = event-data() -> ()  [unwired: 7 out]
        n254 = Negate(x="Phase adj. (GI)") -> (-x=w326:i16)
        n255 = Select(t=w326, s="+ phase (GI)", f="Phase adj. (GI)") -> (s? t:f=w325:i16)
        n256 = Or(x="+ phase (GI)", y="- phase (GI)") -> (x .or. y?=w321:bool)
        n257 = xnode "Read/Write Control"("FPGA VI Reference In"=w328, "error in"=w327, "Phase count adjustment (GI)"=w325) -> ("FPGA VI Reference Out"=w323:T17, "error out"=w324:errorcluster)
        n258 = xnode "Read/Write Control"("FPGA VI Reference In"=w323, "error in"=w324, "+ phase (GI)"=w321) -> ("error out"=w322:errorcluster)  [unwired: 1 out]
      }
      event "Phase adj. (GI) 2", "+ phase (GI) 2", "- phase (GI) 2": Value Change {
        n259 = event-data() -> ()  [unwired: 7 out]
        n260 = Negate(x="Phase adj. (GI) 2") -> (-x=w337:i16)
        n261 = Select(t=w337, s="+ phase (GI) 2", f="Phase adj. (GI) 2") -> (s? t:f=w336:i16)
        n262 = Or(x="+ phase (GI) 2", y="- phase (GI) 2") -> (x .or. y?=w332:bool)
        n263 = xnode "Read/Write Control"("FPGA VI Reference In"=w339, "error in"=w338, "Phase count adjustment (GI) 2"=w336) -> ("FPGA VI Reference Out"=w334:T17, "error out"=w335:errorcluster)
        n264 = xnode "Read/Write Control"("FPGA VI Reference In"=w334, "error in"=w335, "+ phase (GI) 2"=w332) -> ("error out"=w333:errorcluster)  [unwired: 1 out]
      }
      event "Phase adj. (Green FB)", "- phase (Green FB)", "+ phase (Green FB)": Value Change {
        n265 = event-data() -> ()  [unwired: 7 out]
        n266 = Negate(x="Phase adj. (Green FB)") -> (-x=w348:i16)
        n267 = Select(t=w348, s="+ phase (Green FB)", f="Phase adj. (Green FB)") -> (s? t:f=w347:i16)
        n268 = Or(x="+ phase (Green FB)", y="- phase (Green FB)") -> (x .or. y?=w343:bool)
        n269 = xnode "Read/Write Control"("FPGA VI Reference In"=w350, "error in"=w349, "Phase count adjustment (Green FB)"=w347) -> ("FPGA VI Reference Out"=w345:T17, "error out"=w346:errorcluster)
        n270 = xnode "Read/Write Control"("FPGA VI Reference In"=w345, "error in"=w346, "+ phase (Green FB)"=w343) -> ("error out"=w344:errorcluster)  [unwired: 1 out]
      }
      event "Invert APD Gate", "APD Gate ON Count", "APD Gate OFF Count", "APD Gate", "APD Integration Time (s)", "APD 1 AO Mult.", "APD 2 AO Mult.": Value Change {
        n271 = event-data() -> ()  [unwired: 7 out]
        n272 = local read "APD Integration Time (s)"() -> (w351:dbl)
        n273 = local read "APD Gate ON Count"() -> (w364:u32)
        n274 = local read "APD Gate OFF Count"() -> (w363:u32)
        n275 = local read "Invert APD Gate"() -> (w365:bool)
        n276 = local read "APD Gate"() -> (w362:enum32{"ON", "OFF", "Interlace"})
        n277 = Multiply(x=w351, y=40000000.0) -> (x*y=w360:dbl)
        n278 = Reciprocal(x=w351) -> (1/x=→"APD Acq Rate (Hz)":dbl)
        n279 = To Unsigned Long Integer(number=w360) -> (unsigned 32bit integer=w359:u32)
        n280 = local read "DMA Update Period (s)"() -> (w352:dbl)
        n281 = Divide(x=w352, y=w351) -> (x/y=w355:dbl)
        n282 = local read "APD 1 AO Mult."() -> (w357:i16)
        n283 = local read "APD 2 AO Mult."() -> (w356:i16)
        n284 = Multiply(x=2.0, y=w355) -> (x*y=w354:dbl)
        n285 = local write "APD Samples/FIFO Acq."(w355) -> ()
        n286 = local write "APD Elements/DMA read"(w354) -> ()
        n287 = xnode "Read/Write Control"("FPGA VI Reference In"=w368, "error in"=w367, "Invert APD Gate"=w365, "APD Gate ON Count"=w364, "APD Gate OFF Count"=w363, "APD Acq Rate Count"=w359, "APD Gate Operating Mode"=w362, "APD 1 AO scale factor"=w357, "APD 2 AO scale factor"=w356) -> ("error out"=w366:errorcluster)  [unwired: 1 out]
      }
      event "GI Frequency, ON count", "Green FB Count", "GI Frequency, OFF count": Value Change {
        n288 = event-data() -> ()  [unwired: 7 out]
        n289 = xnode "Read/Write Control"("FPGA VI Reference In"=w374, "error in"=w372, "Green interlace ON count"="GI Frequency, ON count", "Green interlace OFF count"="GI Frequency, OFF count", "Green interlace ON count 2"="GI Frequency, ON count", "Green interlace OFF count 2"="GI Frequency, OFF count", "Green FB Count"="Green FB Count") -> ("error out"=w373:errorcluster)  [unwired: 1 out]
      }
      event "Number of F/B Scans (AOD)", "Scan Speed (nm/s)", "Scan BD", "Initial delta (MHz)", "Step Size (nm)", "Scan Range (nm)": Value Change {
        w431 = 123.0  # AOM cal (nm/MHz)
        n290 = event-data() -> ()  [unwired: 7 out]
        n291 = local read "AOM X Cal (nm/MHz)"() -> (w411:dbl)
        n292 = local read item#-1() -> ()  [unwired: 1 out]
        n293 = local read item#-1() -> ()  [unwired: 1 out]
        n294 = local read item#-1() -> (w421)
        n295 = local read item#-1() -> (w419)
        n296 = Negate(x="Scan Range (nm)") -> (-x=w389:dbl)
        n297 = Divide(x=w389, y=w411) -> (x/y=w393:dbl)
        n298 = Select(t=w421, s="Scan BD", f=w419) -> ()  [unwired: 1 out]
        n299 = Select(s="Scan BD") -> (s? t:f=w422:dbl)  [unwired: 2 in]
        n300 = Unbundle By Name() -> ()  [unwired: 1 in, 2 out]
        n301 = Add(x=w393, y=w422) -> (x+y=w425:dbl)
        n302 = Divide(x=w389, y="Step Size (nm)") -> (x/y=w408:dbl)
        n303 = Divide(x="Step Size (nm)", y=w411) -> (x/y=w417:dbl)
        n304 = Absolute Value(x=w408) -> (abs(x)=w392:dbl)
        n305 = Sign(1:w389) -> (0:w390:dbl)
        n306 = In Range and Coerce(x=w425) -> (coerced(x)=w424:dbl, In Range?=w426:bool)  [unwired: 2 in]
        n307 = To Unsigned Quad Integer(1:w392) -> (0:w407:u64)
        "Scan steps (AOD)" <- w407
        n308 = call "IR AOM freq to word.vi"("Frequency In (MHz)"=w417) -> ("Frequency Word Out (double)"=w414:dbl)
        n309 = Multiply(x=w390, y=w414) -> (x*y=w391:dbl)
        n310 = Subtract(x=w425, y=w424) -> (x-y=w423:dbl)
        n311 = To Quad Integer(1:w391) -> (0:w413:i64)
        "Incr. int (AOD)" <- w413
        n312 = Subtract(x=w393, y=w423) -> (x-y=w412:dbl)
        "Scan Range (MHz)" <- w412
        n313 = Select(t=w393, s=w426, f=w412) -> (s? t:f=w427:dbl)
        n314 = Multiply(x=w412, y=w411) -> (x*y=w410:dbl)
        n315 = Decrement(x=w407) -> (x-1=w453:u64)
        n316 = Negate(x=w410) -> (-x=w406:dbl)
        n317 = local write "Scan Range (nm)"(w406) -> ()
        n318 = Divide(x=w427, y=w453) -> (x/y=w416:dbl)
        "Scan Increment (MHz)" <- w416
        n319 = call "IR AOM freq to word.vi"("Frequency In (MHz)"=w416) -> ("Frequency Word Out (double)"=w415:dbl)
        n320 = Divide(x="Step Size (nm)", y="Scan Speed (nm/s)") -> (x/y=w403:dbl)
        n321 = To Quad Integer(1:w415) -> ()  [unwired: 1 out]
        n322 = local read "Number Interlace Sets"() -> (w387:u8)
        n323 = local read "AI Count (ticks)"() -> (w388:u32)
        n324 = local read "Total Counts (ticks)"() -> (w386:u32)
        n325 = local read "# Samples/trap"() -> (w418:u32)
        n326 = Multiply(x=w388, y=w387) -> (x*y=w385:u32)
        n327 = Divide(x=w386, y=w385) -> (x/y=w384:dbl)
        n328 = Select(s="Scan BD") -> (s? t:f=w450:dbl)  [unwired: 2 in]
        "Initial freq. (MHz)" <- w450
        n329 = Add(x=w427, y=w450) -> (x+y=→"Final freq. (MHz)":dbl)
        n330 = Divide(x=w386, y=40000000.0) -> (x/y=w402:dbl)
        n331 = Divide(x=w403, y=w402) -> (x/y=w401:dbl)
        n332 = To Unsigned Quad Integer(1:w401) -> (0:w376:u64)
        n333 = Quotient & Remainder(x=w376, y=u64 2) -> (x-y*floor(x/y)=w380:u64)  [unwired: 1 out]
        n334 = Equal?(x=w380, y=u64 0) -> (x = y?=w378:bool)
        n335 = Decrement(x=w376) -> (x-1=w377:u64)
        n336 = Select(t=w376, s=w378, f=w377) -> (s? t:f=w375:u64)
        "Cycles/step (AOD)" <- w375
        n337 = xnode "Read/Write Control"("FPGA VI Reference In"=w461, "error in"=w460, "Scan steps"=w407, "Number of scans"="Number of F/B Scans (AOD)", "Cycles per step"=w375, "Scan freq.  increment"=w413, "Scan BD"="Scan BD") -> ("error out"=w459:errorcluster)  [unwired: 1 out]
        n338 = Multiply(x=w407, y=w375) -> (x*y=w454:u64)
        n339 = Multiply(x=w454, y=u64 2) -> (x*y=w383:u64)
        n340 = Multiply(x=w384, y=w383) -> (x*y=w382:dbl)
        "Data points/scan (f/b)" <- w382
        n341 = Multiply(x=w382, y="Number of F/B Scans (AOD)") -> (x*y=w457:dbl)
        "Data points/scans" <- w457
        n342 = Divide(x=w457, y=w418) -> (x/y=→"N sets should be saved":dbl)
        n343 = Multiply(x=w454, y=w402) -> (x*y=w400:dbl)
        "Time/Scan (s) (AOD)" <- w400
        n344 = Select(t=w427, s="Scan BD", f=0.0) -> (s? t:f=w451:dbl)
        n345 = Select(t=0.0, s="Scan BD", f=w427) -> (s? t:f=w447:dbl)
        n346 = Add(x=w447) -> (x+y=w445:dbl)  [unwired: 1 in]
        n347 = Add(y=w451) -> (x+y=w446:dbl)  [unwired: 1 in]
        n348 = Multiply(x=w400, y=2.0) -> (x*y=w399:dbl)
        n349 = local read item#-1() -> ()  [unwired: 1 out]
        n350 = local read item#-1() -> ()  [unwired: 1 out]
        n351 = Multiply(x=w399, y="Number of F/B Scans (AOD)") -> (x*y=w396:dbl)
        n352 = Divide(x=w396, y=60.0) -> (x/y=→"Time to Finish All (min)":dbl)
        n353 = Add(x="Trap 2 Bead Size (nm)", y="Trap 1 Bead Size (nm)") -> (x+y=w435:dbl)
        n354 = local read "Initial delta (MHz)"() -> (w432:dbl)
        n355 = Divide(x=w435, y=2.0) -> (x/y=w429:dbl)
        n356 = Subtract(x=w445) -> (x-y=w443:dbl)  [unwired: 1 in]
        n357 = Subtract(x=w446) -> (x-y=w444:dbl)  [unwired: 1 in]
        n358 = Square(x=w443) -> (x^2=w442:dbl)
        n359 = Square(x=w444) -> (x^2=w441:dbl)
        n360 = Add(x=w441, y=w442) -> (x+y=w440:dbl)
        n361 = Square Root(x=w440) -> (sqrt(x)=w439:dbl)
        "Final delta (MHz)" <- w439
        n362 = Multiply(x=w431, y=w439) -> (x*y=w438:dbl)
        n363 = Multiply(x=w432, y=w431) -> (x*y=w430:dbl)
        n364 = Subtract(x=w430, y=w429) -> (x-y=→"Initial sep (nm)":dbl)
        n365 = Subtract(x=w438, y=w429) -> (x-y=→"Final sep (nm)":dbl)
      }
      event #31 (no event record) {
        n366 = event-data() -> ()  [unwired: 7 out]
        n367 = case shown="True" {
          selector: _ -> [_ _]
          frame False {
          }
          frame True {
            (unwired) 65.0 ("Value (Signaling)")
          }
        }
      }
      event "Phase increment trap 1", "Swap F1 and F2", "Freq switch delay", "Amp switch delay", "Phase increment trap 2", "RF phase reset before cycles", "Phase offset method": Value Change {
        n368 = event-data() -> ()  [unwired: 7 out]
        n369 = local read "Amp switch delay"() -> (w466:u16)
        n370 = local read "Phase increment trap 1"() -> (w465:fxp<+/-,64,32>)
        n371 = local read "Freq switch delay"() -> (w468:u16)
        n372 = local read "Phase increment trap 2"() -> (w464:fxp<+/-,64,32>)
        n373 = local read "RF phase reset before cycles"() -> (w463:bool)
        n374 = local read "Swap F1 and F2"() -> (w467:bool)
        n375 = local read "Phase offset method"() -> (w462:u8)
        n376 = xnode "Read/Write Control"("FPGA VI Reference In"=w471, "error in"=w470, "BD 1 Delay (ticks)"=w468, "Swap F1 and F2"=w467, "Amp switch delay"=w466, "Phase Trap 1"=w465, "Phase Trap 2"=w464, "RF phase reset before cycles"=w463, "Phase offset method"=w462) -> ("error out"=w469:errorcluster)  [unwired: 1 out]
      }
      event "Number of scans (MCL)", "Scan Range (V)\n(of steps)", "2D or 1D Scan", "N APD Samp/step", "Fast Scan Dir", "Continuous MCL Scanning": Value Change {
        w472 = 32767.0 ("y")
        n377 = event-data() -> ()  [unwired: 7 out]
        n378 = Select(s="2D or 1D Scan", f="Number of scans (MCL)") -> (s? t:f=w477:u64)  [unwired: 1 in]
        n379 = Decrement() -> (x-1=w491:dbl)  [unwired: 1 in]
        n380 = Divide(x="Scan Range (V)\n(of steps)", y=w491) -> (x/y=w490:dbl)
        "Desired Scan Incr (V)" <- w490
        n381 = local read "APD Integration Time (s)"() -> (w484:dbl)
        n382 = Multiply(x=w490, y=w472) -> (x*y=w499:dbl)
        n383 = Divide(x=w499, y=10.0) -> (x/y=w489:dbl)
        "Desired incr (int)" <- w489
        n384 = local read "Update Count (MCL)"() -> (w495:u32)
        n385 = Round Toward -Infinity(1:w489) -> (0:w498:dbl)
        n386 = To Word Integer(number=w498) -> (16bit integer=w475:i16)
        "Actual Incr. int (MCL)" <- w475
        n387 = Multiply(x=w484, y=40000000.0) -> (x*y=w496:dbl)
        n388 = Divide(x=w496, y=w495) -> (x/y=w494:dbl)
        n389 = Multiply(x=i16 10, y=w475) -> (x*y=w473:i16)
        n390 = Multiply(x="N APD Samp/step", y=w494) -> (x*y=w493:dbl)
        "Cycles/step (MCL)" <- w493
        n391 = Divide(x=w473, y=w472) -> ()  [unwired: 1 out]
        n392 = Multiply(x="N APD Samp/step") -> (x*y=w486:dbl)  [unwired: 1 in]
        n393 = local read "APD Samples/FIFO Acq."() -> (w483:dbl)
        n394 = Multiply(x=w486, y=u64 2) -> (x*y=w485:dbl)
        "Data points/scan (f+b)" <- w485
        n395 = Multiply(x=w485, y=w477) -> (x*y=w502:dbl)
        "Data points/scans (MCL)" <- w502
        n396 = Multiply(x=w484, y=w485) -> (x*y=w478:dbl)
        "Time/f+b scan (s) (MCL)" <- w478
        n397 = Divide(x=w502, y=w483) -> (x/y=→"N sets should be saved (MCL)":dbl)
        n398 = Multiply(x=w478, y=w477) -> (x*y=→"Total Time (s) 2":dbl)
        n399 = Not(x="Fast Scan Dir") -> (.not. x?=w481:bool)
        n400 = xnode "Read/Write Control"("FPGA VI Reference In"=w506, "error in"=w505, "Number of scans (MCL)"=w477, "Cycles per step (MCL)"=w493, "Scan freq.  increment (MCL)"=w475, "1D or 2D Scan?"="2D or 1D Scan", "MCL Scan Axis"=w481, "Cont. Scan (MCL)"="Continuous MCL Scanning") -> ("error out"=w504:errorcluster)  [unwired: 1 in, 1 out]
      }
      event "Read Cal": Value Change {
        w539 = 1000.0 ("y")
        w527 = T16."big-endian, network order" ("byte order (0:big-endian, network order)")
        w528 = -1 ("count (1)")
        n401 = event-data() -> ()  [unwired: 7 out]
        n402 = local read "Save file name"() -> (w557:path)
        n403 = local write "Read Cal"(FALSE ("Read Cal")) -> ()
        n404 = Strip Path(path=w557) -> (stripped path=w556:path)  [unwired: 1 out]
        n405 = Path To String(path=w556) -> (string=w537:string)
        n406 = Concatenate Strings(w537, "\\current.off" ("string")) -> (w535:string)
        n407 = Concatenate Strings(w537, "\\current.cal" ("string")) -> (w554:string)
        n408 = String To Path(string=w554) -> (path=w553:path)
        n409 = String To Path(string=w535) -> (path=w534:path)
        n410 = Open/Create/Replace File(file path (use dialog)=w553, operation (0:open)=T15."open", access (0:read/write)=enum16{"read/write", "read-only", "write-only"}."read-only") -> (refnum out=w560:refnum<file>, error out=w549:errorcluster)  [unwired: 1 in, 3 out]
        n411 = Deny Access(4:w549, 7:w560) -> (0:w548:errorcluster, 3:w552:refnum<file>)  [unwired: 1 out]
        n412 = Open/Create/Replace File(file path (use dialog)=w534, operation (0:open)=T15."open", access (0:read/write)=enum16{"read/write", "read-only", "write-only"}."read-only") -> (refnum out=w531:refnum<file>)  [unwired: 1 in, 4 out]
        n413 = Deny Access(7:w531) -> (3:w529:refnum<file>)  [unwired: 1 in, 2 out]
        n414 = Read from Binary File(5:0.0, 8:w548, 9:w527, 10:w528, 11:w552) -> (0:w547:errorcluster, 2:w545:dbl[], 3:w550:refnum<file>)  [unwired: 2 out]
        n415 = Array To Cluster(array=w545) -> (cluster=w544:T19)
        n416 = Unbundle(w544) -> ("[0]"=w518:dbl, "[1]"=w516:dbl, "[2]"=w517:dbl, "[3]"=w515:dbl, "[4]"=w543:dbl, "[5]"=w542:dbl)
        n417 = Close File(refnum=w550, error in=w547) -> (error out=→"Read cal error":errorcluster)  [unwired: 1 out]
        n418 = Multiply(x=w542, y=w539) -> (x*y=w540:dbl)
        n419 = local write "T2 kappa_x (pN/nm)"(w515) -> ()
        n420 = local write "T1 kappa_x (pN/nm)"(w517) -> ()
        n421 = local write "T1 alpha_x (nm/V)"(w518) -> ()
        n422 = local write "T2 alpha_x (nm/V)"(w516) -> ()
        n423 = Read from Binary File(5:0.0, 9:w527, 10:w528, 11:w529) -> (2:w523:dbl[], 3:w526:refnum<file>)  [unwired: 1 in, 3 out]
        n424 = Multiply(x=w543, y=w539) -> (x*y=w541:dbl)
        n425 = local write "T1 offset_x (mV)"(w541) -> ()
        n426 = local write "T2 offset_x (mV)"(w540) -> ()
        n427 = Close File(refnum=w526) -> ()  [unwired: 1 in, 2 out]
        n428 = Array Subset(array=w523, index=3) -> (w521:dbl[])  [unwired: 1 in]
        n429 = Index Array(array=w523, index=0) -> (element=→"Offset file step size":dbl)
        n430 = Multiply(x=w518, y=w517) -> (x*y=w513:dbl)
        n431 = Multiply(x=w516, y=w515) -> (x*y=w514:dbl)
        n432 = Divide(x=w514, y=w513) -> (x/y=w508:dbl)
        n433 = Decimate 1D Array(w521) -> (w511:dbl[], w512:dbl[])  [unwired: 1 out]
        n434 = property on="B factor" class="DigNum (strict)"("Val(Sgnl)"=w508) -> ()  [unwired: 2 in, 2 out]
        n435 = Bundle By Name(cluster="Offset Values", "Trap 1X offset"=w511, "Trap 2X offset"=w512) -> (w519:T8)
        n436 = Multiply(x=w512, y=w508) -> (x*y=w510:dbl[])
        n437 = Subtract(x=w511, y=w510) -> (x-y=w509:dbl[])
        n438 = local write "Offset Values"(w519) -> ()
        n439 = case shown="True" "Auto read offset\ncorrection" {
          tunnel: w509 -> [_ w561]
          frame False {
          }
          frame True {
            n440 = property on="Setpoint offset\nCorrection values" class="Arr (strict)"("Val(Sgnl)"=w561) -> ()  [unwired: 2 in, 2 out]
          }
        }
      }
      event "Abort MCL Scan": Value Change {
        n441 = event-data() -> ()  [unwired: 7 out]
        n442 = local write "MCL Scanning"(FALSE ("MCL Scanning")) -> ()
        n443 = xnode "Read/Write Control"("FPGA VI Reference In"=w566, "error in"=w565, "Abort scan (MCL)"="Abort MCL Scan") -> ("error out"=w564:errorcluster)  [unwired: 1 out]
      }
      event "Update Count (MCL)": Value Change {
        n444 = event-data() -> ()  [unwired: 7 out]
        n445 = xnode "Read/Write Control"("FPGA VI Reference In"=w570, "error in"=w569, "MCL count"="Update Count (MCL)") -> ("error out"=w568:errorcluster)  [unwired: 1 out]
      }
      event "Phase adjust (MCL)", "+ phase (MCL)", "- phase (MCL)": Value Change {
        n446 = event-data() -> ()  [unwired: 7 out]
        n447 = Negate(x="Phase adjust (MCL)") -> (-x=w579:i16)
        n448 = Select(t=w579, s="- phase (MCL)", f="Phase adjust (MCL)") -> (s? t:f=w577:i16)
        n449 = Or(x="- phase (MCL)", y="+ phase (MCL)") -> (x .or. y?=w572:bool)
        n450 = xnode "Read/Write Control"("FPGA VI Reference In"=w581, "error in"=w580, "Phase count adjustment (MCL)"=w577) -> ("FPGA VI Reference Out"=w573:T17, "error out"=w574:errorcluster)
        n451 = xnode "Read/Write Control"("FPGA VI Reference In"=w573, "error in"=w574, "+ phase (MCL)"=w572) -> ("error out"=w571:errorcluster)  [unwired: 1 out]
      }
      event "Abort AOD Scan": Value Change {
        n452 = event-data() -> ()  [unwired: 7 out]
        n453 = flat-sequence {
          tunnel: w586 -> [w592]
          tunnel: w585 -> [w591]
          tunnel: [w590] -> w583
          tunnel: [w587] -> w582
          tunnel: [w603] -> w584
          tunnel: w583 -> [w603]
          tunnel: w582 -> [w602]
          frame #0 {
            (unwired) FALSE
            n454 = local read "Save scans"() -> (w588:bool)
            n455 = xnode "Read/Write Control"("FPGA VI Reference In"=w592, "error in"=w591, "Abort scan"="Abort AOD Scan") -> ("FPGA VI Reference Out"=w587:T17, "error out"=w590:errorcluster)
            n456 = case shown="True" w588 {
              frame False {
              }
              frame True {
                (unwired) TRUE
                n457 = local read item#-1() -> ()  [unwired: 1 in]
              }
            }
            n458 = local read item#-1() -> ()  [unwired: 1 in]
          }
          frame #1 {
            n459 = xnode "Read/Write Control"("FPGA VI Reference In"=w602) -> ("BD1 Frequency Out 1"=w593:u64)  [unwired: 1 in, 2 out]
            n460 = To Double Precision Float(number=w593) -> (double precision float=w599:dbl)
            n461 = Multiply(x=49125000.0, y=6.0) -> (x*y=w598:dbl)
            n462 = Multiply(x=w599, y=w598) -> (x*y=w596:dbl)
            n463 = Scale By Power Of 2(n=-48, x=w596) -> (x*2^n=w595:dbl)
            n464 = Divide(x=w595, y=1000000.0) -> ()  [unwired: 1 out]
          }
        }
      }
      event "Continuous AOD Scanning": Value Change {
        n465 = event-data() -> ()  [unwired: 7 out]
        n466 = xnode "Read/Write Control"("FPGA VI Reference In"=w607, "error in"=w606, "Cont. Scan"="Continuous AOD Scanning") -> ("error out"=w605:errorcluster)  [unwired: 1 out]
      }
      event "Index": Value Change {
        n467 = event-data() -> ()  [unwired: 7 out]
        n468 = call "Create new save file.vi"("Insert"="", "Ext"=".dat" ("string"), "Index In"="Index") -> ("Path Out"=→"Save file name":path, "Index Out"=w608:dbl)
        "Save index" <- w608
        n469 = local write "Index"(w608) -> ()
      }
      event #41 (no event record) {
        w621 = 10.0 ("y")
        w620 = 32767.0 ("y")
        n470 = event-data() -> ()  [unwired: 7 out]
        n471 = local read item#-1() -> ()  [unwired: 1 out]
        n472 = local read item#-1() -> ()  [unwired: 1 out]
        n473 = Multiply(y=w620) -> (x*y=w617:dbl)  [unwired: 1 in]
        n474 = Multiply(y=w620) -> (x*y=w619:dbl)  [unwired: 1 in]
        n475 = Divide(x=w617, y=w621) -> (x/y=w616:dbl)
        n476 = Divide(x=w619, y=w621) -> (x/y=w618:dbl)
        n477 = To Word Integer(number=w616) -> (16bit integer=w622:i16)
        n478 = To Word Integer(number=w618) -> (16bit integer=w623:i16)
        n479 = xnode "Read/Write Control"("FPGA VI Reference In"=w615, "error in"=w614, "AO1 (Y)"=w622, "AO2 (X)"=w623) -> ("error out"=w613:errorcluster)  [unwired: 1 out]
      }
      event "Inject Top:": Value Change {
        n480 = event-data() -> ()  [unwired: 7 out]
        n481 = disable-structure shown="Enabled" {
          disable-tunnel: "Inject Top:" -> [w625 w665]
          frame Disabled {
            n482 = local read "Chemyx Syringe Pump Serial Port"() -> (w626:refnum<visa-resource-name>)
            n483 = local read "Pump write delay (ms)"() -> (w627:dbl)
            n484 = case shown="True" w625 {
              tunnel: w627 -> [w633 w647]
              tunnel: w626 -> [w630 w646]
              frame False {
                n485 = flat-sequence {
                  tunnel: w630 -> [w634]
                  tunnel: [w634] -> w631
                  tunnel: w633 -> [_]
                  tunnel: [w637] -> w632
                  tunnel: w631 -> [w637]
                  tunnel: w632 -> [w638]
                  tunnel: [w638] -> w628
                  tunnel: [w640] -> w629
                  tunnel: w628 -> [w640]
                  tunnel: w629 -> [w642]
                  frame #0 {
                    n486 = call "Write to pump.vi"("string"="enter pump1", "VISA resource name"=w634) -> ()  [unwired: 1 out]
                  }
                  frame #1 {
                    n487 = Wait (ms)(milliseconds to wait="Pump pause delay (ms)") -> ()  [unwired: 1 out]
                  }
                  frame #2 {
                    n488 = call "Write to pump.vi"("string"="stop", "VISA resource name"=w638) -> ()  [unwired: 1 out]
                  }
                  frame #3 {
                    n489 = Wait (ms)(milliseconds to wait=u32 500) -> ()  [unwired: 1 out]
                  }
                  frame #4 {
                    n490 = call "Write to pump.vi"("string"="stop", "VISA resource name"=w642) -> ()  [unwired: 1 out]
                  }
                }
              }
              frame True {
                n491 = flat-sequence {
                  tunnel: w646 -> [w656]
                  tunnel: w647 -> [w651]
                  tunnel: w647 -> [w658]
                  tunnel: w646 -> [w659]
                  tunnel: [w659] -> w644
                  tunnel: [w661] -> w645
                  tunnel: w644 -> [w661]
                  tunnel: w645 -> [w663]
                  frame #0 {
                    n492 = local read "All Pump Parameters"() -> (w650:T3)
                    n493 = Unbundle By Name(w650) -> ("Pump 1"=w657:T20)
                    n494 = call "Set pump parameters.vi"("Pump write delay (ms)"=w651, "Volume (uL)"="Ch 2 Inject Volume (uL)", "Rate (uL/h)"="Ch 1 Inject Rate (ul/h)", "Units"=4.0, "Pump #"=1.0, "Pump Parameters In"=w657, "VISA resource name"=w656) -> ("Pump Parameters Out"=w649:T20)  [unwired: 3 in]
                    n495 = Bundle By Name(cluster=w650, "Pump 1"=w649) -> (w648:T3)
                    n496 = local write "All Pump Parameters"(w648) -> ()
                  }
                  frame #1 {
                    n497 = Wait (ms)(milliseconds to wait=w658) -> ()  [unwired: 1 out]
                  }
                  frame #2 {
                    n498 = call "Write to pump.vi"("string"="start", "VISA resource name"=w659) -> ()  [unwired: 1 out]
                  }
                  frame #3 {
                    n499 = Wait (ms)(milliseconds to wait=u32 500) -> ()  [unwired: 1 out]
                  }
                  frame #4 {
                    n500 = call "Write to pump.vi"("string"="start", "VISA resource name"=w663) -> ()  [unwired: 1 out]
                  }
                }
              }
            }
          }
          frame Enabled {
            n501 = call "hamilton_controller.vi"("Open?"=w665, "valve"=enum16{"A", "B", "C", "D", "ALL"}."B", "action"=T14."MOVE VALVE") -> ()  [unwired: 8 in, 1 out]
          }
        }
      }
      event "Main:": Value Change {
        n502 = event-data() -> ()  [unwired: 7 out]
        n503 = disable-structure shown="Disabled" {
          disable-tunnel: "Main:" -> [_ w709]
          frame Disabled {
            n504 = local read "Pump write delay (ms)"() -> (w670:dbl)
            n505 = case shown="False" w671 {
              tunnel: w670 -> [w677 w691]
              tunnel: "Chemyx Syringe Pump Serial Port" -> [w674 w690]
              frame False {
                n506 = flat-sequence {
                  tunnel: w674 -> [w678]
                  tunnel: [w678] -> w675
                  tunnel: w677 -> [_]
                  tunnel: [w681] -> w676
                  tunnel: w675 -> [w681]
                  tunnel: w676 -> [w682]
                  tunnel: [w682] -> w672
                  tunnel: [w684] -> w673
                  tunnel: w672 -> [w684]
                  tunnel: w673 -> [w686]
                  frame #0 {
                    n507 = call "Write to pump.vi"("string"="enter pump3", "VISA resource name"=w678) -> ()  [unwired: 1 out]
                  }
                  frame #1 {
                    n508 = local read "Pump pause delay (ms)"() -> (w680:u32)
                    n509 = Wait (ms)(milliseconds to wait=w680) -> ()  [unwired: 1 out]
                  }
                  frame #2 {
                    n510 = call "Write to pump.vi"("string"="stop", "VISA resource name"=w682) -> ()  [unwired: 1 out]
                  }
                  frame #3 {
                    n511 = Wait (ms)(milliseconds to wait=u32 0) -> ()  [unwired: 1 out]
                  }
                  frame #4 {
                    n512 = call "Write to pump.vi"("string"="stop", "VISA resource name"=w686) -> ()  [unwired: 1 out]
                  }
                }
              }
              frame True {
                n513 = flat-sequence {
                  tunnel: w690 -> [w700]
                  tunnel: w691 -> [w695]
                  tunnel: w691 -> [w702]
                  tunnel: w690 -> [w703]
                  tunnel: [w703] -> w688
                  tunnel: [w706] -> w689
                  tunnel: w688 -> [w706]
                  tunnel: w689 -> [w707]
                  frame #0 {
                    n514 = local read "All Pump Parameters"() -> (w694:T3)
                    n515 = Unbundle By Name(w694) -> ("Pump 3"=w701:T20)
                    n516 = call "Set pump parameters.vi"("Pump write delay (ms)"=w695, "Volume (uL)"="Ch 3 Inject Volume (uL)", "Rate (uL/h)"="Ch 3 Inject Rate (ul/h)", "Units"=4.0, "Pump #"=3.0, "Pump Parameters In"=w701, "VISA resource name"=w700) -> ("Pump Parameters Out"=w693:T20)  [unwired: 3 in]
                    n517 = Bundle By Name(cluster=w694, "Pump 3"=w693) -> (w692:T3)
                    n518 = local write "All Pump Parameters"(w692) -> ()
                  }
                  frame #1 {
                    n519 = Wait (ms)(milliseconds to wait=w702) -> ()  [unwired: 1 out]
                  }
                  frame #2 {
                    n520 = call "Write to pump.vi"("string"="start", "VISA resource name"=w703) -> ()  [unwired: 1 out]
                  }
                  frame #3 {
                    n521 = Wait (ms)(milliseconds to wait=u32 500) -> ()  [unwired: 1 out]
                  }
                  frame #4 {
                    n522 = call "Write to pump.vi"("string"="start", "VISA resource name"=w707) -> ()  [unwired: 1 out]
                  }
                }
              }
            }
          }
          frame Enabled {
            n523 = call "hamilton_controller.vi"("Open?"=w709, "valve"=enum16{"A", "B", "C", "D", "ALL"}."A", "action"=T14."MOVE VALVE") -> ()  [unwired: 8 in, 1 out]
          }
        }
      }
      event "Inject Valve B": Value Change {
        n524 = event-data() -> ()  [unwired: 7 out]
        n525 = disable-structure shown="Enabled" {
          disable-tunnel: "Inject Valve B" -> [w713 w733]
          frame Disabled {
            n526 = local read "Pump write delay (ms)"() -> (w715:dbl)
            n527 = flat-sequence {
              tunnel: w714 -> [w728]
              tunnel: w715 -> [w724]
              tunnel: w713 -> [_]
              tunnel: w715 -> [w730]
              tunnel: w714 -> [w731]
              frame #0 {
                n528 = local read "All Pump Parameters"() -> (w723:T3)
                n529 = Multiply(x=60.0, y="Flush Center Ch Rate (ul/m)") -> (x*y=w720:dbl)
                n530 = Unbundle By Name(w723) -> ("Pump 2"=w729:T20)
                n531 = call "Set pump parameters.vi"("Pump write delay (ms)"=w724, "Volume (uL)"="Flush Center Ch Volume (uL)", "Rate (uL/h)"=w720, "Units"=3.0, "Pump #"=2.0, "Pump Parameters In"=w729, "VISA resource name"=w728) -> ("Pump Parameters Out"=w722:T20)  [unwired: 3 in]
                n532 = Bundle By Name(cluster=w723, "Pump 2"=w722) -> (w721:T3)
                n533 = local write "All Pump Parameters"(w721) -> ()
                n534 = Add(x="Flush Center Ch Volume (uL)", y="Total Volume\nFlushed (uL)") -> (x+y=w717:dbl)
                n535 = local write "Total Volume\nFlushed (uL)"(w717) -> ()
              }
              frame #1 {
                n536 = Wait (ms)(milliseconds to wait=w730) -> ()  [unwired: 1 out]
              }
              frame #2 {
                n537 = call "Write to pump.vi"("string"="start", "VISA resource name"=w731) -> ()  [unwired: 1 out]
              }
            }
            n538 = local read "Chemyx Syringe Pump Serial Port"() -> (w714:refnum<visa-resource-name>)
          }
          frame Enabled {
            n539 = call "hamilton_controller.vi"("Open?"=w733, "valve"=enum16{"A", "B", "C", "D", "ALL"}."B", "action"=T14."MOVE VALVE") -> ()  [unwired: 8 in, 1 out]
          }
        }
      }
      event "Inject Bottom": Value Change {
        n540 = event-data() -> ()  [unwired: 7 out]
        n541 = call "hamilton_controller.vi"("Open?"="Inject Bottom", "valve"=enum16{"A", "B", "C", "D", "ALL"}."C", "action"=T14."MOVE VALVE") -> ()  [unwired: 8 in, 1 out]
      }
      event "Shunt:": Value Change {
        n542 = event-data() -> ()  [unwired: 7 out]
        n543 = call "hamilton_controller.vi"("Open?"="Shunt:", "valve"=enum16{"A", "B", "C", "D", "ALL"}."D", "action"=T14."MOVE VALVE") -> ()  [unwired: 8 in, 1 out]
      }
      event "Flip Green Filter": Value Change {
        n544 = event-data() -> ()  [unwired: 7 out]
        n545 = local write "Flip Green Filter"("Flip Green Filter") -> ()
        n546 = flat-sequence {
          tunnel: w749 -> [w754]
          tunnel: w748 -> [w753]
          tunnel: [w751] -> w746
          tunnel: [w750] -> w745
          tunnel: [w756] -> w744
          tunnel: w746 -> [w756]
          tunnel: [w755] -> w743
          tunnel: w745 -> [w755]
          tunnel: w744 -> [w760]
          tunnel: w743 -> [w759]
          tunnel: [w758] -> w747
          frame #0 {
            n547 = xnode "Read/Write Control"("FPGA VI Reference In"=w754, "error in"=w753, "Green Filter Flipper"=TRUE) -> ("FPGA VI Reference Out"=w751:T17, "error out"=w750:errorcluster)
          }
          frame #1 {
            n548 = Wait (ms)(milliseconds to wait=u32 100) -> ()  [unwired: 1 out]
          }
          frame #2 {
            n549 = xnode "Read/Write Control"("FPGA VI Reference In"=w760, "error in"=w759, "Green Filter Flipper"=FALSE) -> ("error out"=w758:errorcluster)  [unwired: 1 out]
          }
        }
      }
      event "Pump 1 contents", "Pump 3 contents": Value Change {
        n550 = event-data() -> ()  [unwired: 7 out]
        n551 = local read "Pump 1 contents"() -> (→"Pump 1 cont disp":string)
        n552 = local read "Pump 3 contents"() -> (→"Pump 3 cont disp":string)
      }
      event "Reset Trap Pos. FB": Value Change {
        n553 = event-data() -> ()  [unwired: 7 out]
        n554 = xnode "Read/Write Control"("FPGA VI Reference In"=w766, "error in"=w765, "Trap Pos. FB Reset"="Reset Trap Pos. FB") -> ()  [unwired: 2 out]
      }
      event "Trap Pos. FB ON": Value Change {
        n555 = event-data() -> ()  [unwired: 7 out]
        n556 = xnode "Read/Write Control"("FPGA VI Reference In"=w781, "error in"=w780) -> ("FPGA VI Reference Out"=w778:T17, "BD1 Frequency Out 1"=w775:u64)  [unwired: 1 out]
        n557 = To Double Precision Float(number=w775) -> (double precision float=w774:dbl)
        n558 = Multiply(x=49125000.0, y=6.0) -> (x*y=w773:dbl)
        n559 = Multiply(x=w774, y=w773) -> (x*y=w771:dbl)
        n560 = Scale By Power Of 2(n=-48, x=w771) -> (x*2^n=w770:dbl)
        n561 = Divide(x=w770, y=1000000.0) -> (x/y=w767:dbl)
        n562 = flat-sequence {
          tunnel: [w784] -> w779
          tunnel: w778 -> [w785]
          tunnel: w775 -> [w783]
          tunnel: "Trap Pos. FB ON" -> [w782]
          tunnel: "Trap Pos. FB ON" -> [w791]
          tunnel: w779 -> [w790]
          tunnel: "Trap Pos. FB ON" -> [w793]
          tunnel: w767 -> [w792]
          frame #0 {
            n563 = case shown="False" w782 {
              tunnel: w785 -> [w788 w789]
              tunnel: [w787 w789] -> w784
              tunnel: w783 -> [w786 _]
              frame False {
                n564 = xnode "Read/Write Control"("FPGA VI Reference In"=w788, "BD 1 Frequency 1"=w786) -> ("FPGA VI Reference Out"=w787:T17)  [unwired: 1 in, 1 out]
              }
              frame True {
              }
            }
          }
          frame #1 {
            n565 = xnode "Read/Write Control"("FPGA VI Reference In"=w790, "Force feedback"=w791) -> ()  [unwired: 1 in, 2 out]
          }
          frame #2 {
            n566 = case shown="False" w793 {
              tunnel: w792 -> [w794 _]
              frame False {
                n567 = Subtract(x=90.0, y=w794) -> ()  [unwired: 1 out]
              }
              frame True {
              }
            }
          }
        }
      }
      event "Diff. FB.", "Trap Pos. FB Gains", "Trap Pos. FB Mult Factor", "Trap Pos. FB Offset Factor", "Trap Pos FB Negate Action", "Trap Pos FB Monitor\nT1 or T2", "Negate Diff?": Value Change {
        n568 = event-data() -> ()  [unwired: 7 out]
        n569 = xnode "Read/Write Control"("FPGA VI Reference In"=w806, "error in"=w805, "Trap pos. FB Range"="Trap Pos. FB Range", "Trap Pos. FB Gains"="Trap Pos. FB Gains", "Trap Pos. FB Mult Factor"="Trap Pos. FB Mult Factor", "Trap Pos. FB Offset Factor"="Trap Pos. FB Offset Factor", "Trap Pos FB Negate Action"="Trap Pos FB Negate Action", "Trap Pos FB Monitor T1 or T2"="Trap Pos FB Monitor\nT1 or T2", "AI1 X Scale"="Trap Pos. AI1 X Pre-scale", "Negate Diff?"="Negate Diff?", "Diff FB Measurement?"="Diff. FB.") -> ()  [unwired: 2 out]
      }
      event "Trap Pos FB SP": Value Change {
        n570 = event-data() -> ()  [unwired: 7 out]
        n571 = xnode "Read/Write Control"("FPGA VI Reference In"=w809, "error in"=w808, "Trap Pos. FB SP"="Trap Pos FB SP") -> ()  [unwired: 2 out]
      }
      event "Simulate stepping": Value Change {
        n572 = event-data() -> ()  [unwired: 7 out]
        n573 = flat-sequence {
          tunnel: w811 -> [w814]
          tunnel: [w813] -> _
          tunnel: w810 -> [w812]
          frame #0 {
            n574 = while {
              tunnel: w814 -> [w834]
              tunnel: [w833] -> w813 mode=indexing
              tunnel: w812 -> [w832]
              i -> [w822]
              stop <- w819 stop-if-true
              w816 = 1000.0
              n575 = Divide(x="Backtrack probability", y=100) -> (x/y=w842:dbl)
              n576 = Random Number (0-1)() -> (number: 0 to 1=w843:dbl)
              n577 = Greater?(x=w843, y=w842) -> (0:w841:bool)
              n578 = Select(t=1, s=w841, f=-1) -> (s? t:f=w838:i32)
              n579 = Multiply(x=w838, y="Step size (nm)") -> (x*y=w836:dbl)
              "Step taken" <- w836
              n580 = local read item#-1() -> ()  [unwired: 1 out]
              n581 = Divide(x=w836, y=168.33) -> (x/y=w818:dbl)
              n582 = local read item#-1() -> ()  [unwired: 1 out]
              n583 = local read item#-1() -> ()  [unwired: 1 out]
              n584 = local read item#-1() -> ()  [unwired: 1 out]
              n585 = Subtract(y=w818) -> ()  [unwired: 1 in, 1 out]
              n586 = local read item#-1() -> ()  [unwired: 1 in]
              n587 = call "set RF board frequency - interlace.vi"("error in"=w834, "FPGA VI Reference In"=w832) -> ("error out"=w833:errorcluster)  [unwired: 8 in, 1 out]
              n588 = local read item#-1() -> ()  [unwired: 1 out]
              n589 = local read item#-1() -> ()  [unwired: 1 out]
              n590 = Subtract() -> (x-y=w831:dbl)  [unwired: 2 in]
              n591 = Subtract() -> (x-y=w830:dbl)  [unwired: 2 in]
              n592 = Square(x=w830) -> (x^2=w828:dbl)
              n593 = Square(x=w831) -> (x^2=w829:dbl)
              n594 = Add(x=w829, y=w828) -> (x+y=w827:dbl)
              n595 = Square Root(x=w827) -> ()  [unwired: 1 out]
              n596 = local read item#-1() -> ()  [unwired: 1 in]
              n597 = property on="Initial delta (MHz)" class="DigNum (strict)" props=["Val(Sgnl)"]() -> ()  [unwired: 3 in, 2 out]
              n598 = Multiply(x="Mean dwell time (s)", y=w816) -> (x*y=w824:dbl)
              n599 = case shown="\"Gamma2\"" "Distribution" {
                tunnel: w824 -> [w847 w851 w854]
                tunnel: [w847 w848 w855] -> w817
                frame "uniform", Default {
                }
                frame "Exponential" {
                  n600 = call-poly <vilib>:"Continuous Random.vi"("b"=w851, "samples"=1) -> ("exp random data"=w849:dbl[])  [unwired: 8 in, 1 out]
                  n601 = Index Array(array=w849) -> (element=w848:dbl)  [unwired: 1 in]
                }
                frame "Gamma2" {
                  w852 = 2.0
                  # "Note: the shape and scale\nparameters of the gamma\nare inverted because LabView..."
                  n602 = Divide(x=w854, y=w852) -> (x/y=w853:dbl)
                  n603 = call-poly <vilib>:"Continuous Random.vi"("c"=w853, "b"=w852, "samples"=1) -> ("gamma random numbers"=w856:dbl[])  [unwired: 7 in, 1 out]
                  n604 = Index Array(array=w856) -> (element=w855:dbl)  [unwired: 1 in]
                }
              }
              n605 = Divide(x=w817, y=w816) -> (x/y=→"Step duration":dbl)
              n606 = To Unsigned Long Integer(number=w817) -> (unsigned 32bit integer=w825:u32)
              n607 = Add(x=w822, y=1) -> (x+y=w821:i32)
              n608 = Wait (ms)(milliseconds to wait=w825) -> ()  [unwired: 1 out]
              n609 = Equal?(x=w821, y="Number of steps") -> (x = y?=w819:bool)
            }
          }
          frame #1 {
            n610 = local write "Simulate stepping"(FALSE) -> ()
          }
        }
      }
      event "Set SP to Reading": Value Change {
        n611 = event-data() -> ()  [unwired: 7 out]
        n612 = local read "Trap Pos FB Monitor\nT1 or T2"() -> (w866:bool)
        n613 = local read "Trap X AI1 (DMA)"() -> (w869:T2)
        n614 = local read "Trap X (AI1)"() -> (w872:T1)
        n615 = Unbundle By Name(w872) -> ("Trap 1"=w871:fxp<+/-,16,1>, "Trap 2"=w870:fxp<+/-,16,1>)
        n616 = Unbundle By Name(w869) -> ("Set 1"=w868:fxp<+/-,16,1>, "Set 2"=w867:fxp<+/-,16,1>)
        n617 = Select(t=w871, s=w866, f=w870) -> (s? t:f=w865:fxp<+/-,16,1>)
        n618 = Select(t=w868, s=w866, f=w867) -> (s? t:f=w864:fxp<+/-,16,1>)
        n619 = Not(x="Set SP Using...") -> (.not. x?=w859:bool)
        n620 = Select(t=w865, s=w859, f=w864) -> (s? t:f=w860:fxp<+/-,16,1>)
        n621 = xnode "Read/Write Control"("FPGA VI Reference In"=w862, "error in"=w861, "Trap Pos. FB SP"=w860) -> ()  [unwired: 2 out]
        n622 = local write "Trap Pos FB SP"(w860) -> ()
      }
      event "Trap Pos. FB Out Scale 2^n": Value Change {
        n623 = event-data() -> ()  [unwired: 7 out]
        n624 = Scale By Power Of 2(n="Trap Pos. FB Out Scale 2^n", x=ext 1.0) -> (x*2^n=w874:ext)
        n625 = property on="Trap Pos. FB Mult Factor" class="DigNum (strict)"("Val(Sgnl)"=w874) -> ()  [unwired: 2 in, 2 out]
      }
      event "Trap Pos FB Int Count": Value Change {
        n626 = event-data() -> ()  [unwired: 7 out]
        n627 = xnode "Read/Write Control"("FPGA VI Reference In"=w879, "error in"=w878, "Trap Pos FB Int Count"="Trap Pos FB Int Count") -> ()  [unwired: 2 out]
      }
      event "Target Force (pN)", "Setpoint offset\nCorrection values", "Raster target force (pN)": Value Change {
        w887 = 2.0
        n628 = event-data() -> ()  [unwired: 7 out]
        n629 = local read "B factor"() -> (w917:dbl)
        n630 = To Fixed-Point(number=w917) -> (fixed-point=w916:fxp<+/-,16,16>)  [unwired: 1 in]
        n631 = xnode "Read/Write Control"("FPGA VI Reference In"=w881, "B factor"=w916) -> ("BD1 Frequency Out 1"=w907:u64)  [unwired: 1 in, 2 out]
        n632 = local read item#-1() -> ()  [unwired: 1 out]
        n633 = local read "Target Force (pN)"() -> (w893:dbl)
        n634 = To Double Precision Float(number=w907) -> (double precision float=w913:dbl)
        n635 = Multiply(x=49125000.0, y=6.0) -> (x*y=w912:dbl)
        n636 = Multiply(x=w913, y=w912) -> (x*y=w910:dbl)
        n637 = Scale By Power Of 2(n=-48, x=w910) -> (x*2^n=w909:dbl)
        n638 = Divide(x=w909, y=1000000.0) -> (x/y=w906:dbl)
        n639 = Subtract(y=w906) -> (x-y=w905:dbl)  [unwired: 1 in]
        n640 = local read "T1 kappa_x (pN/nm)"() -> (w894:dbl)
        n641 = local read "T1 alpha_x (nm/V)"() -> (w895:dbl)
        n642 = local read "Negate offset difference"() -> (w896:bool)
        n643 = local read "Offset file step size"() -> (w904:dbl)
        n644 = Multiply(x="Raster target force (pN)", y=w887) -> (x*y=w886:dbl)
        n645 = Multiply(x=w893, y=w887) -> (x*y=w892:dbl)
        n646 = local read "Setpoint offset\nCorrection values"() -> (w901:dbl[])
        n647 = Divide(x=w905, y=w904) -> (x/y=w903:dbl)
        n648 = Select(t=-1, s=w896, f=1) -> (s? t:f=w897:i32)
        n649 = To Long Integer(number=w903) -> (32bit integer=w902:i32)
        n650 = Multiply(x=w895, y=w894) -> (x*y=w885:dbl)
        n651 = Divide(x=w892, y=w885) -> (x/y=w891:dbl)
        n652 = Index Array(array=w901, index=w902) -> (element=w900:dbl)
        n653 = Divide(x=w886, y=w885) -> (x/y=w884:dbl)
        n654 = Multiply(x=w897, y=w900) -> (x*y=w883:dbl)
        n655 = Add(x=w891, y=w883) -> (x+y=w890:dbl)
        n656 = Add(x=w884, y=w883) -> (x+y=w882:dbl)
        n657 = To Fixed-Point(number=w882) -> (fixed-point=w880:fxp<+/-,16,1>)  [unwired: 1 in]
        n658 = To Fixed-Point(number=w890) -> (fixed-point=w889:fxp<+/-,16,1>)  [unwired: 1 in]
        n659 = property on="Trap Pos FB SP" class="DigNum (strict)"("Val(Sgnl)"=w889) -> ()  [unwired: 2 in, 2 out]
        n660 = xnode "Read/Write Control"("FPGA VI Reference In"=w881, "Raster setpoint"=w880) -> ()  [unwired: 1 in, 2 out]
      }
      event "Read setpoint correction\nfile": Value Change {
        n661 = event-data() -> ()  [unwired: 7 out]
        n662 = local write "Read setpoint correction\nfile"(FALSE) -> ()
        n663 = Open/Create/Replace File(file path (use dialog)="Setpoint correction\noffset file", operation (0:open)=T15."open", access (0:read/write)=enum16{"read/write", "read-only", "write-only"}."read-only") -> (refnum out=w942:refnum<file>)  [unwired: 1 in, 4 out]
        n664 = Deny Access(7:w942) -> (3:w940:refnum<file>)  [unwired: 1 in, 2 out]
        n665 = Read from Binary File(5:0.0, 9:T16."big-endian, network order" ("byte order (0:big-endian, network order)"), 10:-1 ("count (1)"), 11:w940) -> (2:w933:dbl[], 3:w939:refnum<file>)  [unwired: 1 in, 3 out]
        n666 = Close File(refnum=w939) -> ()  [unwired: 1 in, 2 out]
        n667 = Index Array(array=w933, index=0) -> (element=w929:dbl)
        n668 = local write "Offset file step size"(w929) -> ()
        n669 = Array Subset(array=w933, index=3) -> (w932:dbl[])  [unwired: 1 in]
        n670 = local read "T1 kappa_x (pN/nm)"() -> (w927:dbl)
        n671 = local read "T1 alpha_x (nm/V)"() -> (w928:dbl)
        n672 = local read "T2 alpha_x (nm/V)"() -> (w926:dbl)
        n673 = local read "T2 kappa_x (pN/nm)"() -> (w925:dbl)
        n674 = Decimate 1D Array(w932) -> (w920:dbl[], w921:dbl[])  [unwired: 1 out]
        n675 = local read "Offset Values"() -> (w931:T8)
        n676 = Multiply(x=w928, y=w927) -> (x*y=w923:dbl)
        n677 = Multiply(x=w926, y=w925) -> (x*y=w924:dbl)
        n678 = Bundle By Name(cluster=w931, "Trap 1X offset"=w920, "Trap 2X offset"=w921) -> (w930:T8)
        n679 = Divide(x=w924, y=w923) -> (x/y=w922:dbl)
        n680 = property on="B factor" class="DigNum (strict)"("Val(Sgnl)"=w922) -> ()  [unwired: 2 in, 2 out]
        n681 = Multiply(x=w921, y=w922) -> (x*y=w919:dbl[])
        n682 = local write "Offset Values"(w930) -> ()
        n683 = Subtract(x=w920, y=w919) -> (x-y=w918:dbl[])
        n684 = property on="Setpoint offset\nCorrection values" class="Arr (strict)"("Val(Sgnl)"=w918) -> ()  [unwired: 2 in, 2 out]
      }
      event "MCL Tracking": Value Change {
        n685 = event-data() -> ()  [unwired: 7 out]
        n686 = case shown="True" "MCL Tracking" {
          frame False {
            n687 = local read "Current MCL (V)"() -> ()  [unwired: 1 out]
            n688 = local read item#-1() -> ()  [unwired: 1 in]
          }
          frame True {
            n689 = local read item#-1() -> ()  [unwired: 1 out]
            n690 = local read item#-1() -> ()  [unwired: 1 out]
          }
        }
      }
      event "Scale intensities": Value Change {
        n691 = event-data() -> ()  [unwired: 7 out]
        n692 = local read "Trap Intensity\nSetpoints (V)"() -> (w950:cluster{"Set 1":dbl, "Set 2":dbl})
        n693 = local read "T1 kappa_x (pN/nm)"() -> (w956:dbl)
        n694 = local read "T2 kappa_x (pN/nm)"() -> (w955:dbl)
        n695 = Unbundle By Name(w950) -> ("Set 1"=w952:dbl, "Set 2"=w951:dbl)
        n696 = case shown="False" "Scale intensities" {
          tunnel: "Scale factor" -> [w966 w978]
          tunnel: "Scale factor" -> [w961 w971]
          tunnel: w956 -> [w968 w977]
          tunnel: w955 -> [w967 w976]
          tunnel: [w964 w975] -> w954
          tunnel: [w965 w974] -> w953
          tunnel: w952 -> [w963 w973]
          tunnel: w951 -> [w962 w972]
          tunnel: [w960 w970] -> w949
          tunnel: [w959 w969] -> w948
          frame False {
            n697 = Divide(x=w968, y=w961) -> (x/y=w964:dbl)
            n698 = Divide(x=w967, y=w966) -> (x/y=w965:dbl)
            n699 = Divide(x=w963, y=w961) -> (x/y=w960:dbl)
            n700 = Divide(x=w962, y=w961) -> (x/y=w959:dbl)
          }
          frame True {
            n701 = Multiply(x=w973, y=w971) -> (x*y=w970:dbl)
            n702 = Multiply(x=w972, y=w971) -> (x*y=w969:dbl)
            n703 = Multiply(x=w977, y=w971) -> (x*y=w975:dbl)
            n704 = Multiply(x=w978, y=w976) -> (x*y=w974:dbl)
          }
        }
        n705 = local write "T2 kappa_x (pN/nm)"(w953) -> ()
        n706 = local write "T1 kappa_x (pN/nm)"(w954) -> ()
        n707 = Bundle By Name(cluster=w950, "Set 1"=w949, "Set 2"=w948) -> (w947:cluster{"Set 1":dbl, "Set 2":dbl})
        n708 = local write "Trap Intensity\nSetpoints (V)"(w947) -> ()
      }
    }
    "error out 2" <- w4
    n709 = node-c288() -> ()  [unwired: 1 in, 1 out]
  }
  n710 = node-c288(w1) -> ()  [unwired: 1 out]
